vi "FW Simulator.vi"() -> ()   [LabVIEW 2015]
uses:
  Type/_RT Command.ctl
  Type/_RT Instrument State.ctl
  State.ctl
  Type/_RT Instrument 2.ctl
  Type/_RT Configuration 2.ctl
  Type/RT Loop Events.ctl
  Type/_RT Parameter.ctl
  Type/_RT Active Ch.ctl
  Type/_RT Expt.ctl
  Type/_Run Mode.ctl
  Type/_RT Mass Range.ctl
  Type/_RT Res Type.ctl
  Type/_RT Startup Options.ctl
  Type/_File Command.ctl
  Type/TCP Packet Info.ctl
  Type/_RT Data.ctl
  RT 9607/_FW_Sim Global.vi
  <vilib>/Utility/config.llb/Read Key (Boolean).vi
  Server/_Server Global.vi
  <vilib>/Utility/config.llb/NI_LVConfig.lvlib
panel:
  in  "Tab Control":enum32{"Page 1", "Page 2"}(tab)
  out "Connected":bool
  out "Command":T1
  out "# Connections":u8
  out "Messages":string="PC Communication Established"
  out "System State":T2
  in  "Stop Button":bool
  out "Remaining Scans":i32
  out "InstrState":T3
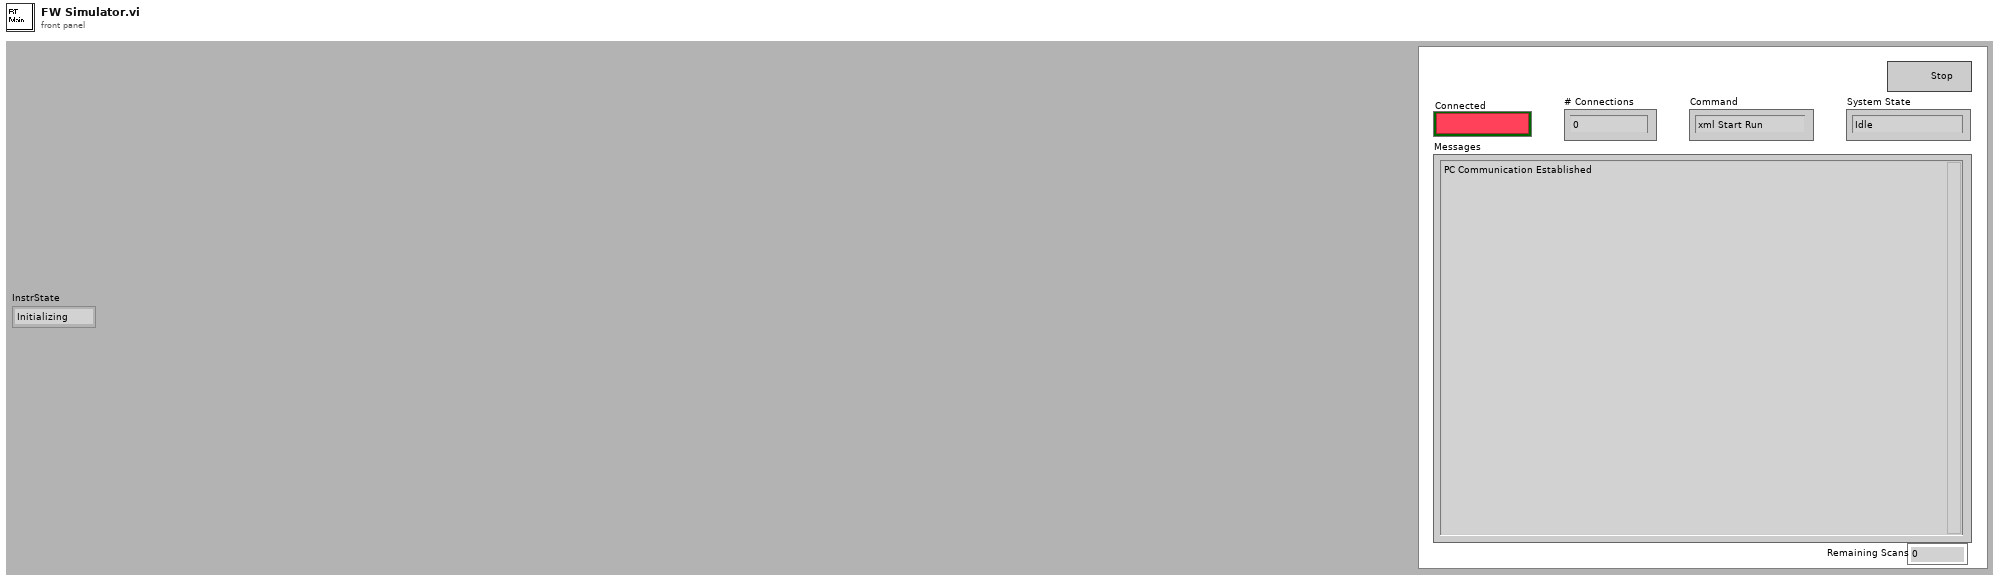
[diagram p1: front panel]
types:
  T1 = typedef "_RT Command.ctl" = enum16{"xml Start Run", "xml Start Actual Run", "xml Stop Run", "xml Runtime Update", "xml Get Status", "xml Get Table", "xml Set Table", "xml Get Configuration", "xml System Status", "xml Set LC Input Logic", "xml Get Data", "xml Get Info", "Start", "StartActualRun", "Stop", "Runtime Update", "Get Data", "Get Info", "Get Status", "Get Param", "Get Config", "Get Table", "Read ADC", "Set Oscillator", "Update Config", "Update Table", "Set All Pol", "Set Pol and DC", "Set Max Mass", "Toggle RP", "Toggle EL", "Set PIC", "Initialize Turbo", "Send Turbo Comm", "Close Turbo", "P1", "P2", "P3", "Send Serial", "Set LC Out", "Get LC In", "Read VAC", "Test Table", "Toggle Power", "Get Startup", "Set Startup", "Get ADC Table", "Set ADC Table", "Get Brief Status", "Get Detail Status", "Auxiliary Update", "Set CC Logics", "Set CC Input Logics", "Ignore Error", "invalid"}
  T2 = typedef "State.ctl" = enum16{"Idle", "Running", "Not Ready", "Fault", "Waiting"}
  T3 = typedef "_RT Instrument State.ctl" = enum16{"Initializing", "Mass Spectrometer is Off", "Starting Up", "Turning Power Off", "Going to Standby", "Roughing Pump Ready", "Turning Turbo Off", "Turbo Startup", "Turbopump Ready", "Checking Vacuum", "Going to Ready", "Ready", "Running", "Source Standby", "Lost Communication", "Shutting Down", "Fault", "24V Standby", "Go to 24V Standby", "Turbopump Ready-Waiting"}
  T4 = typedef "_RT Instrument 2.ctl" = cluster{"Table":T5[], "Instrument":string[]}
  T5 = typedef "_RT Configuration 2.ctl" = cluster{"Name":string, "Ch#":u8, "Min":dbl, "Max":dbl, "Def+":dbl, "Def-":dbl, "Offset":dbl, "Slope":dbl, "Type":u8, "Description":string, "SettleT":dbl}
  T6 = typedef "_RT Parameter.ctl" = cluster{"RunMode":i32, "Initial Ch":T7[], "Sync":u8, "Expt":T8[], "EqTime(mS)":i32}
  T7 = typedef "_RT Active Ch.ctl" = cluster{"Start":i32, "Step":i32, "ChID":i32}
  T8 = typedef "_RT Expt.ctl" = cluster{"StartT(mS)":i32, "#Cycles":i32, "Scan Type":T9, "PauseT(uS)":i32, "Polarity":u8, "DelayT(mS)":i32, "Active Ch":T7[], "Mass Range":T10[]}
  T9 = typedef "_Run Mode.ctl" = enum16{"MRM (Q1/Q2)", "Q1 Scan", "Q1 SRM", "Q2 Scan", "Q2 SRM", "Product Scan", "Precursor Scan", "Neutral Loss", "Neutral Gain"}
  T10 = typedef "_RT Mass Range.ctl" = cluster{"Steps":i32, "Dwell(uS)":i32, "Resolution Type":T11, "Ramping Ch":T7[]}
  T11 = typedef "_RT Res Type.ctl" = u16
  T12 = typedef "RT Loop Events.ctl" = enum16{"Initialize", "Wait for Connection", "Wait for Command", "Send Reply"}
  T13 = cluster{"Rt Loop Events":T12, "Connection ID":refnum<k5>, "Parameter":T6, "Message Data":string, "Data Array":i32[], "Sequence Number":i32, "Command":T1, "error":errorcluster, "Msgs":string}
  T14 = typedef "_RT Startup Options.ctl" = cluster{"Door":bool, "Curtain":bool, "Pressure":bool, "Turbo":bool, "SysPoll":bool, "GasFlag":bool}
  T15 = typedef "_File Command.ctl" = enum16{"No Command", "Open", "Open Read", "Write", "Get Spectrum", "Close"}
  T16 = enum16{"big-endian, network order", "native, host order", "little-endian"}
  T17 = typedef "TCP Packet Info.ctl" = cluster{"Packet Signature":string, "Sequence Number":i32, "Command":T1, "Data Message Size":u32, "Data Message Size":string, "Data Message":string, "Error Message Size":u32, "Error Message Size":string, "Error Message":string, "Checksum":u32, "Error Message":errorcluster, "Command ID":string}
  T18 = typedef "_RT Data.ctl" = cluster{"Info":string, "Data Array":i32[], "error out":errorcluster}
  T19 = typedef "NI_LVConfig.lvlib/Config Data RefNum.ctl" = refnum<k1>
  T20 = typedef "_XML Lens.ctl" = cluster{"Value":dbl, "ChID":u8}
  T21 = typedef "_Server Method.ctl" = cluster{"RunMode":i32, "Sync":u8, "Expt":T22[], "EqTime(mS)":i32, "TuneParam":T7[]}
  T22 = typedef "_XML Expt.ctl" = cluster{"StartT(mS)":i32, "#Cycles":i32, "PauseT(uS)":i32, "ScanType":i32, "Polarity":u8, "FixedMass":dbl, "DelayT(mS)":i32, "Active Ch":T20[], "Mass Range":T23[]}
  T23 = typedef "_Mass Range Property.ctl" = cluster{"Start":dbl, "Stop":dbl, "Step Size":dbl, "Steps":i32, "Dwell":dbl, "Parameters":T24[], "Res":T11}
  T24 = typedef "_Mass Range Parameters.ctl" = cluster{"Name":string, "Ch#":u8, "StartV":dbl, "StopV":dbl, "StepV":dbl, "Index":u8}
  T25 = enum32{"Invalid", "Standard", "Closed", "Hidden", "Minimized", "Maximized"}
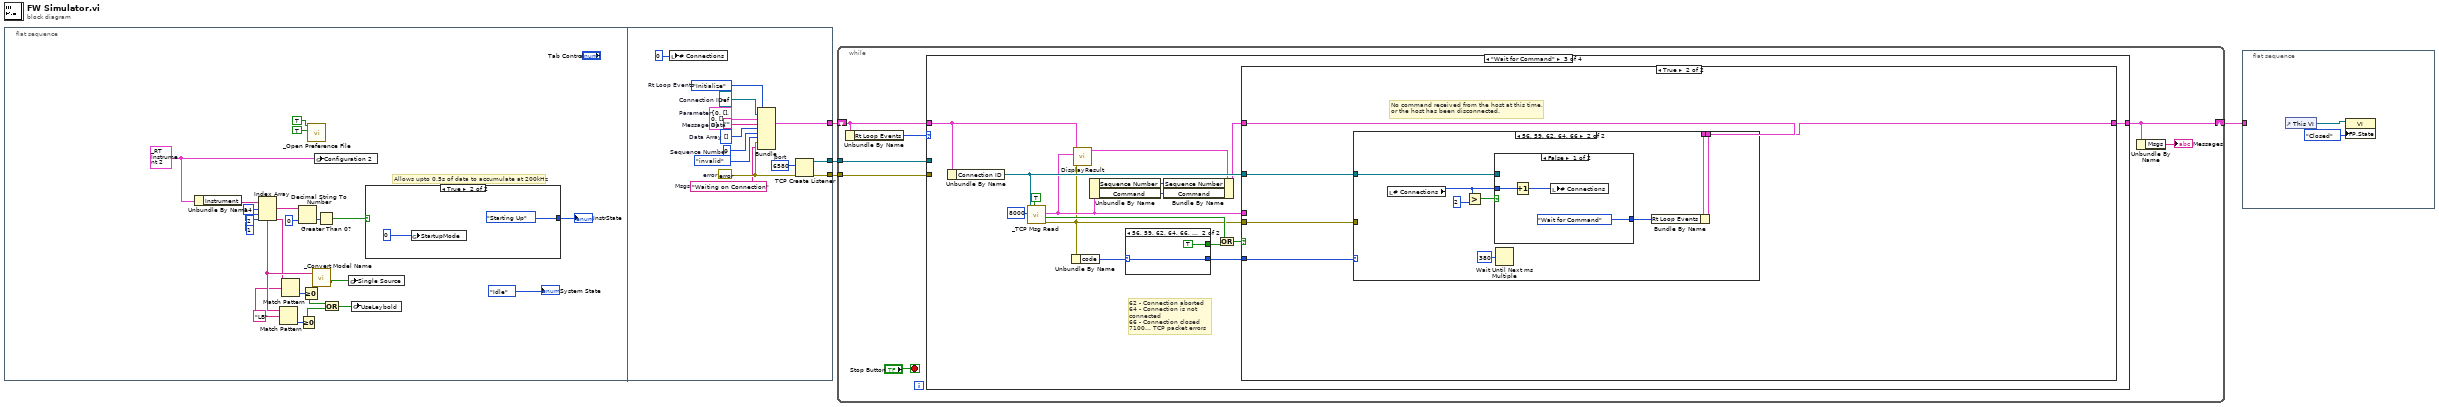
[diagram p0: block diagram]
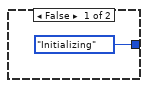
[diagram p2: hidden frame]
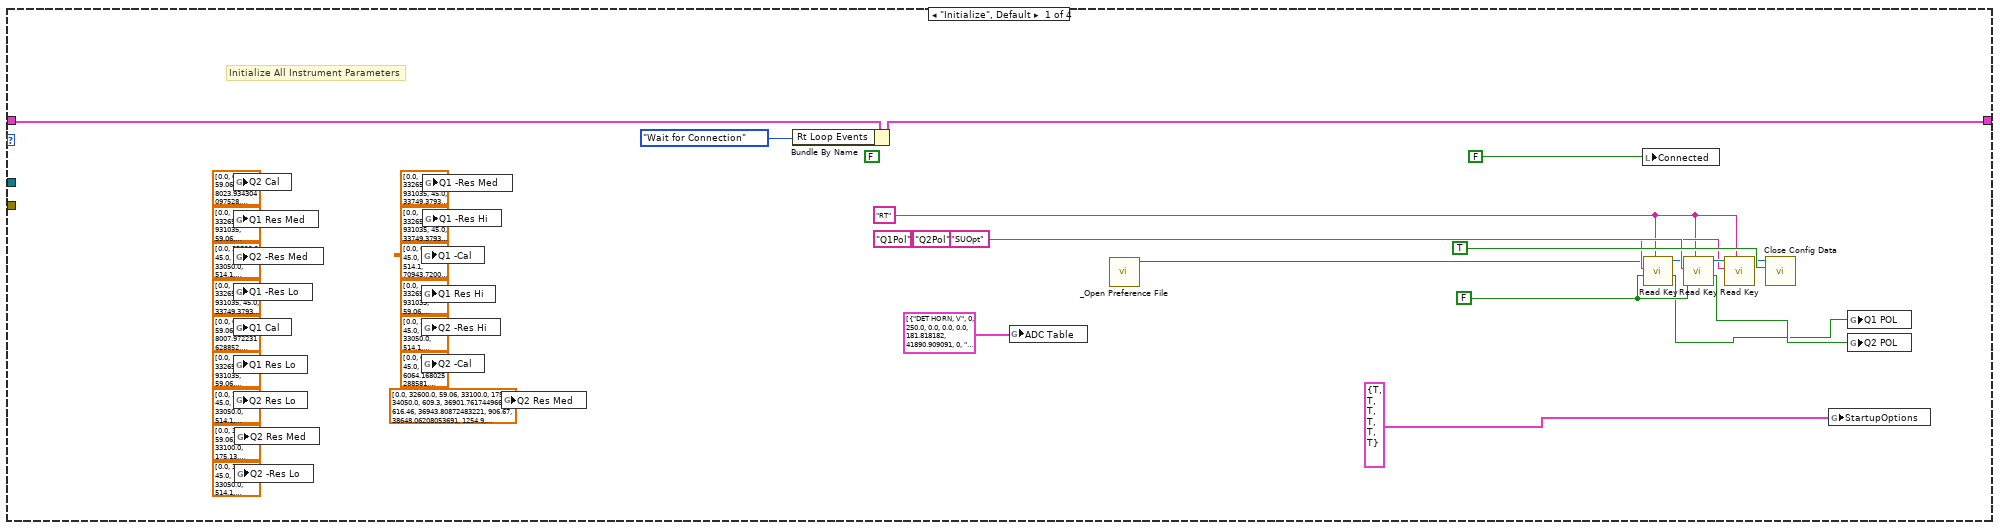
[diagram p3: hidden frame]
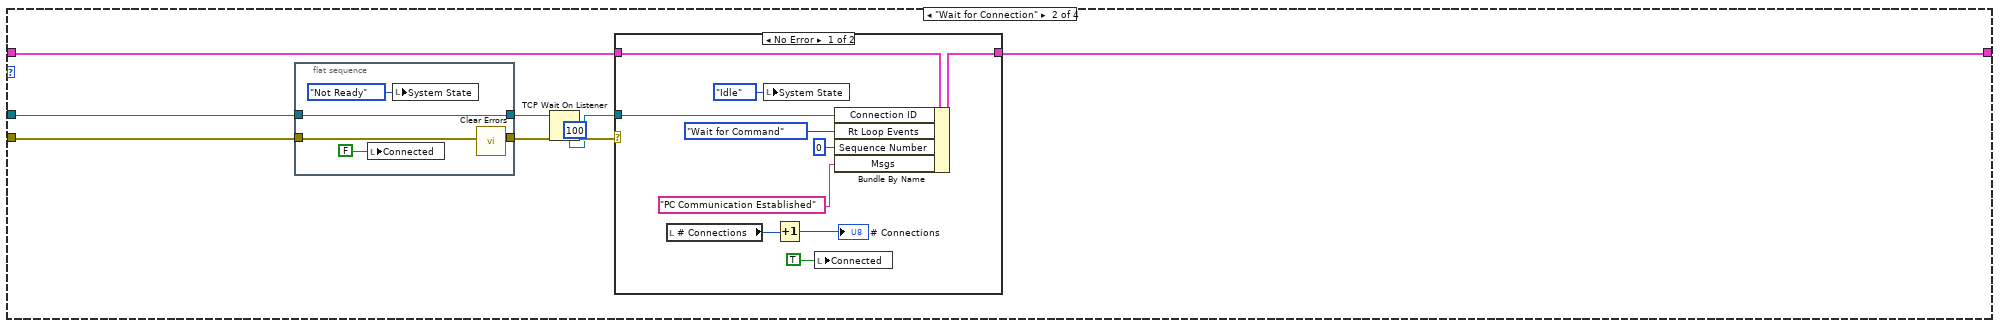
[diagram p4: hidden frame]
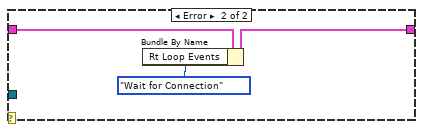
[diagram p5: hidden frame]
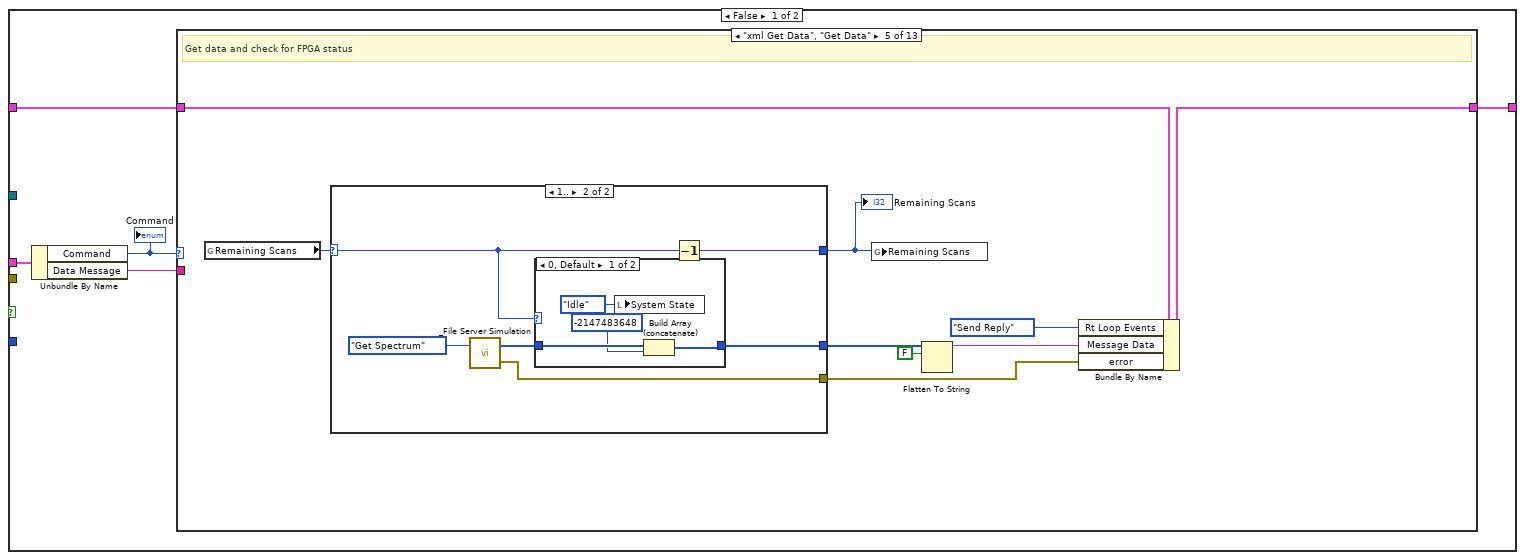
[diagram p6: hidden frame]
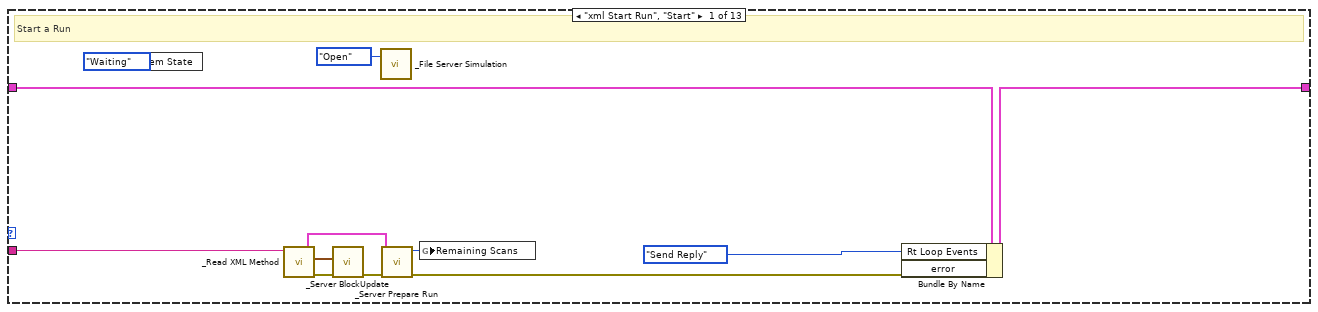
[diagram p7: hidden frame]
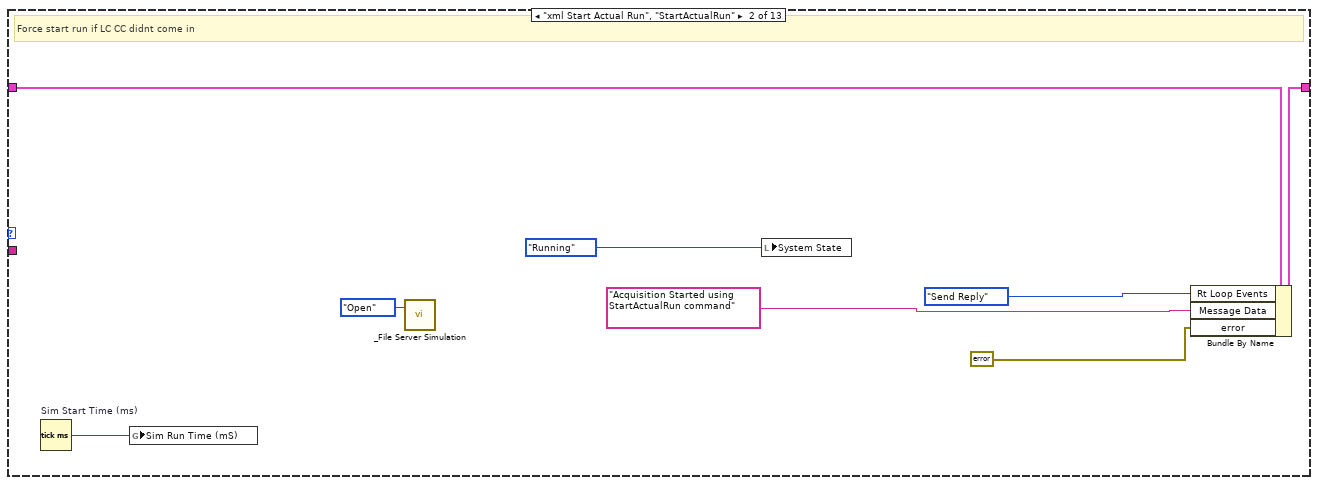
[diagram p8: hidden frame]
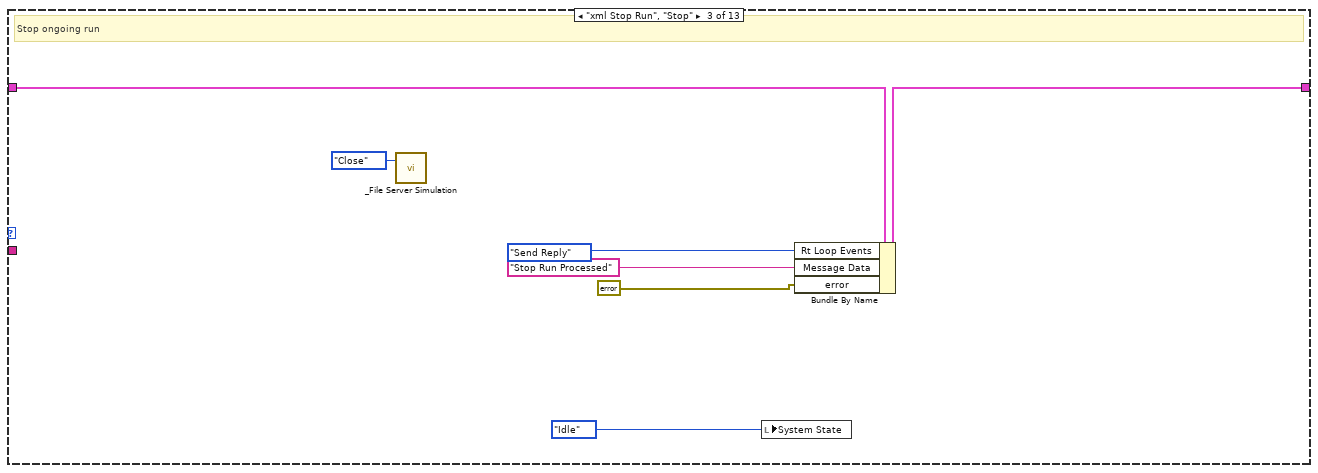
[diagram p9: hidden frame]
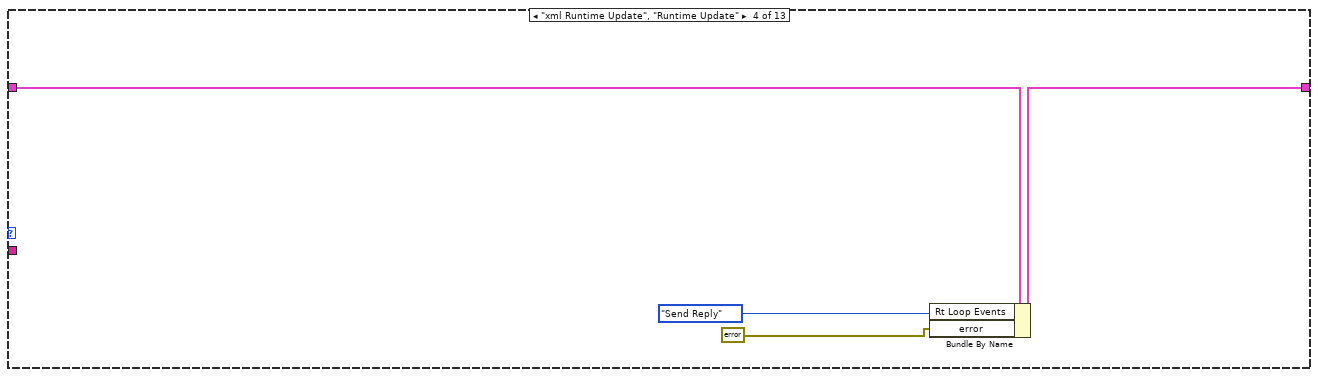
[diagram p10: hidden frame]
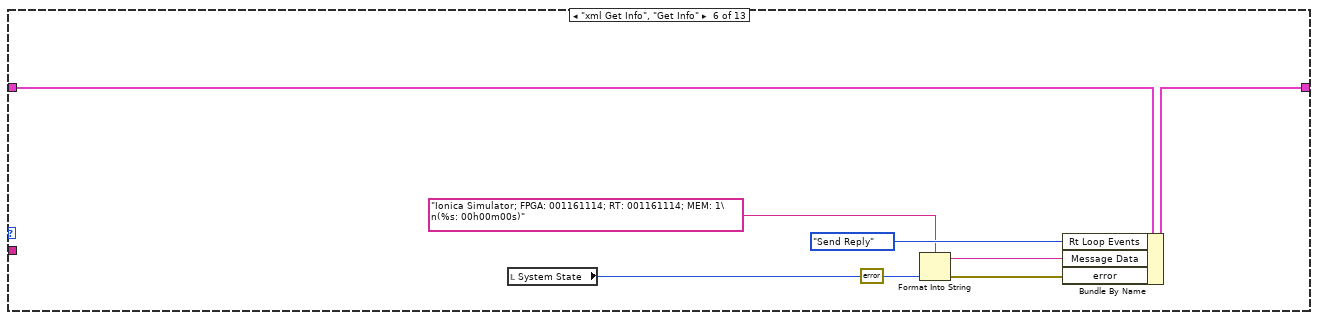
[diagram p13: hidden frame]
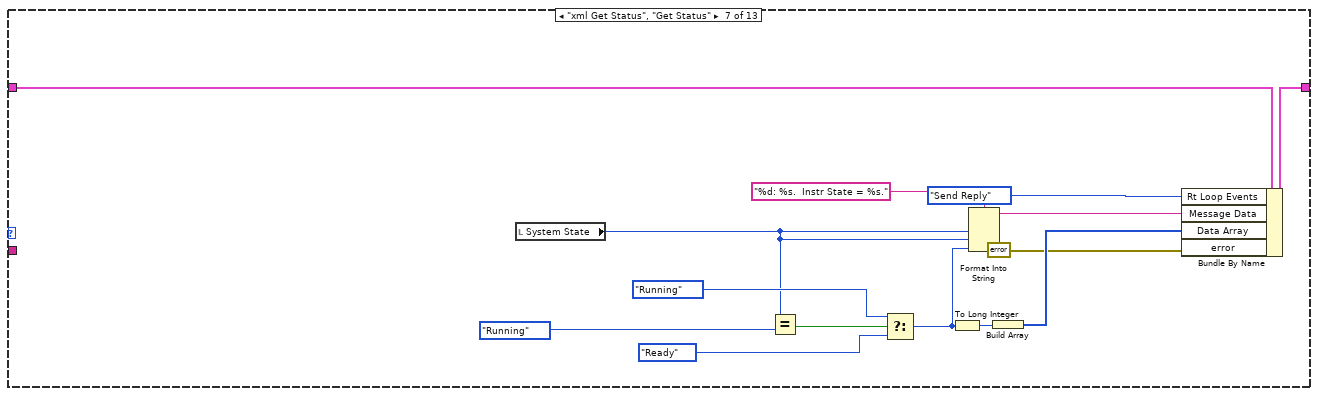
[diagram p14: hidden frame]
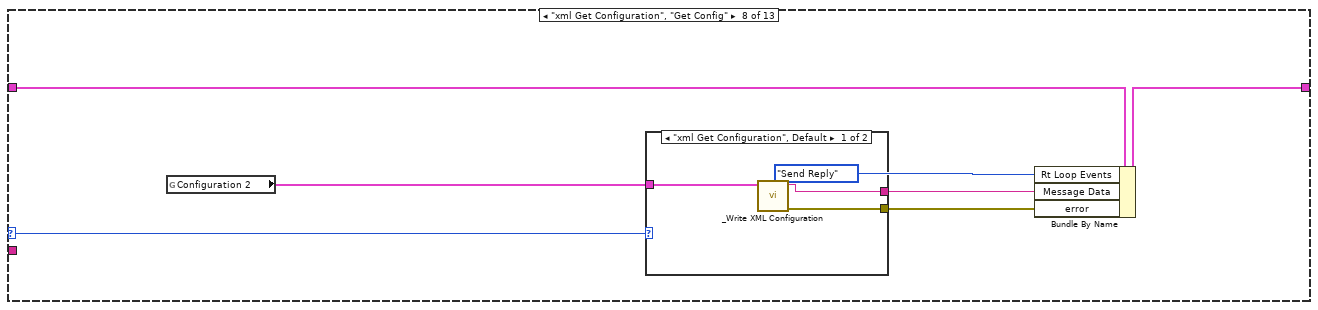
[diagram p15: hidden frame]
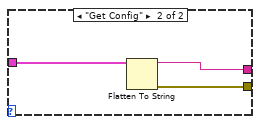
[diagram p16: hidden frame]
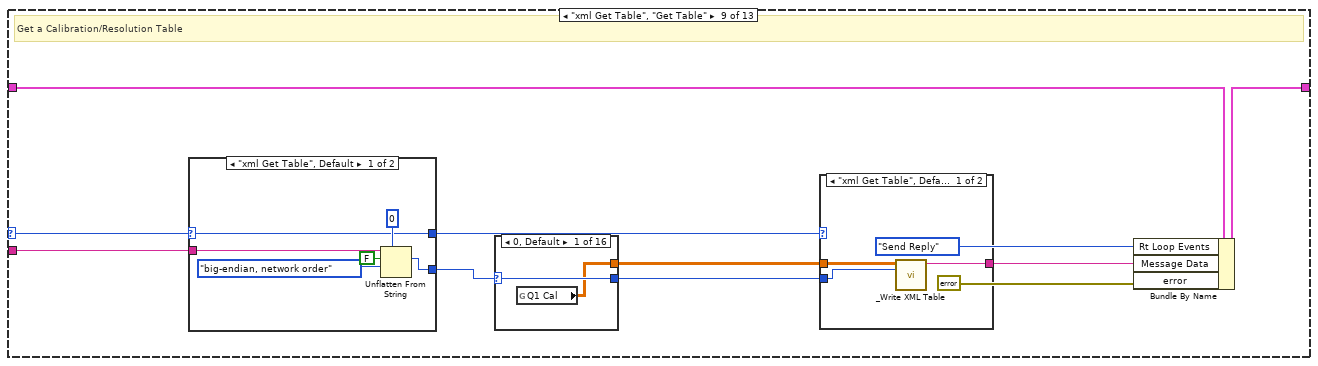
[diagram p17: hidden frame]
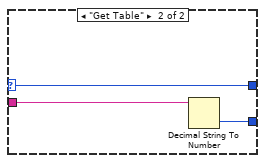
[diagram p18: hidden frame]
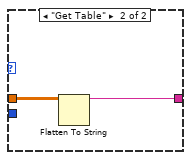
[diagram p19: hidden frame]
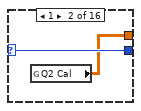
[diagram p20: hidden frame]
diagram:
  n1 = flat-sequence {
    tunnel: [w41] -> w4
    tunnel: [w37] -> w3
    tunnel: [w34] -> w2
    frame #0 {
      w5 = T4 {"Table"=[{"Name"="Q1 RF", "Ch#"=1, "Min"=0.0, "Max"=1500.0, "Def+"=0.0, "Def-"=0.0, "Offset"=0.0, "Slope"=218.45, "Type"=64, "Description"="Quadrupole 1 RF", "SettleT"=5.0}, {"Name"="Q1 DC", "Ch#"=4, "Min"=0.0, "Max"=1500.0, "Def+"=600.0, "Def-"=600.0, "Offset"=0.0, "Slope"=218.45, "Type"=64, "Description"="Quadrupole 1 DC", "SettleT"=5.0}, {"Name"="Q1 RR", "Ch#"=7, "Min"=0.0, "Max"=65535.0, "Def+"=32768.0, "Def-"=32768.0, "Offset"=32768.0, "Slope"=1.0, "Type"=64, "Description"="Quadrupole 1 PW", "SettleT"=5.0}, {"Name"="Q2 RF", "Ch#"=2, "Min"=0.0, "Max"=1500.0, "Def+"=0.0, "Def-"=0.0, "Offset"=0.0, "Slope"=218.45, "Type"=64, "Description"="Quadrupole 2 RF", "SettleT"=5.0}, {"Name"="Q2 DC", "Ch#"=5, "Min"=0.0, "Max"=1500.0, "Def+"=600.0, "Def-"=600.0, "Offset"=0.0, "Slope"=218.45, "Type"=64, "Description"="Quadrupole 2 DC", "SettleT"=5.0}, {"Name"="Q2 RR", "Ch#"=9, "Min"=0.0, "Max"=65535.0, "Def+"=32768.0, "Def-"=32768.0, "Offset"=32743.0, "Slope"=1.0, "Type"=64, "Description"="Quadrupole 2 PW", "SettleT"=5.0}, {"Name"="M1 RF", "Ch#"=3, "Min"=0.0, "Max"=500.0, "Def+"=0.0, "Def-"=0.0, "Offset"=0.0, "Slope"=14.7, "Type"=6, "Description"="Multipole 1 RF", "SettleT"=5.0}, {"Name"="EV", "Ch#"=20, "Min"=-200.0, "Max"=200.0, "Def+"=0.0, "Def-"=0.0, "Offset"=32768.0, "Slope"=-65.7, "Type"=7, "Description"="Entrance Voltage", "SettleT"=5.0}, {"Name"="ED", "Ch#"=21, "Min"=-400.0, "Max"=400.0, "Def+"=0.0, "Def-"=0.0, "Offset"=32768.0, "Slope"=-131.0, "Type"=7, "Description"="Not Used 1", "SettleT"=5.0}, {"Name"="M1", "Ch#"=19, "Min"=-400.0, "Max"=400.0, "Def+"=0.0, "Def-"=0.0, "Offset"=32775.0, "Slope"=-65.60000000000001, "Type"=7, "Description"="Multipole 1", "SettleT"=5.0}, {"Name"="L1", "Ch#"=18, "Min"=-400.0, "Max"=400.0, "Def+"=0.0, "Def-"=0.0, "Offset"=32764.0, "Slope"=-65.89999999999999, "Type"=7, "Description"="Multipole Lens 1", "SettleT"=5.0}, {"Name"="M2", "Ch#"=22, "Min"=-400.0, "Max"=400.0, "Def+"=0.0, "Def-"=0.0, "Offset"=32768.0, "Slope"=-66.0, "Type"=7, "Description"="Multipole 2", "SettleT"=5.0}, {"Name"="L2", "Ch#"=11, "Min"=-400.0, "Max"=400.0, "Def+"=0.0, "Def-"=0.0, "Offset"=32768.0, "Slope"=-65.92, "Type"=7, "Description"="Multipole Lens 2", "SettleT"=5.0}, {"Name"="PF", "Ch#"=12, "Min"=-400.0, "Max"=400.0, "Def+"=-16.0, "Def-"=16.0, "Offset"=32768.00000000001, "Slope"=-65.8, "Type"=7, "Description"="Prefilter 1", "SettleT"=5.0}, {"Name"="Q1", "Ch#"=6, "Min"=-150.0, "Max"=150.0, "Def+"=-1.0, "Def-"=1.0, "Offset"=32755.0, "Slope"=-131.3, "Type"=11, "Description"="Quadrupole 1", "SettleT"=5.0}, {"Name"="CC L1", "Ch#"=13, "Min"=-400.0, "Max"=400.0, "Def+"=0.0, "Def-"=0.0, "Offset"=32768.00000000001, "Slope"=-65.8, "Type"=7, "Description"="Collision Cell Lens 1", "SettleT"=5.0}, {"Name"="CC L2", "Ch#"=14, "Min"=-400.0, "Max"=400.0, "Def+"=-100.0, "Def-"=100.0, "Offset"=32768.00000000001, "Slope"=-65.8, "Type"=7, "Description"="Collision Cell Lens 2", "SettleT"=5.0}, {"Name"="CC", "Ch#"=23, "Min"=-400.0, "Max"=400.0, "Def+"=-50.0, "Def-"=50.0, "Offset"=32735.141073657927, "Slope"=-65.71785268414482, "Type"=7, "Description"="Collision Energy", "SettleT"=5.0}, {"Name"="CC AF", "Ch#"=10, "Min"=-400.0, "Max"=400.0, "Def+"=50.0, "Def-"=-50.0, "Offset"=32768.00000000001, "Slope"=-65.8, "Type"=7, "Description"="Axial Field", "SettleT"=5.0}, {"Name"="CC L3", "Ch#"=15, "Min"=-400.0, "Max"=400.0, "Def+"=-52.5, "Def-"=52.5, "Offset"=32735.10888610764, "Slope"=-65.7822277847309, "Type"=7, "Description"="Collision Cell Lens 3", "SettleT"=5.0}, {"Name"="CC L4", "Ch#"=16, "Min"=-400.0, "Max"=400.0, "Def+"=-72.5, "Def-"=72.5, "Offset"=32768.0, "Slope"=-65.7, "Type"=7, "Description"="Collision Cell Lens 4", "SettleT"=5.0}, {"Name"="Q2", "Ch#"=8, "Min"=-150.0, "Max"=150.0, "Def+"=-54.0, "Def-"=54.0, "Offset"=32756.0, "Slope"=-131.3, "Type"=11, "Description"="Quadrupole 2", "SettleT"=5.0}, {"Name"="ID", "Ch#"=17, "Min"=-400.0, "Max"=400.0, "Def+"=-100.0, "Def-"=100.0, "Offset"=32768.00000000001, "Slope"=-65.8, "Type"=7, "Description"="Detector Deflector", "SettleT"=5.0}, {"Name"="DISC", "Ch#"=32, "Min"=10.0, "Max"=2000.0, "Def+"=20.0, "Def-"=20.0, "Offset"=-5.0, "Slope"=1.23, "Type"=18, "Description"="Discriminator", "SettleT"=10.0}, {"Name"="DV", "Ch#"=34, "Min"=0.0, "Max"=3500.0, "Def+"=2000.0, "Def-"=2000.0, "Offset"=0.0, "Slope"=0.4104084321475626, "Type"=18, "Description"="Detector Voltage", "SettleT"=10.0}, {"Name"="DET horn", "Ch#"=200, "Min"=0.0, "Max"=5500.0, "Def+"=5500.0, "Def-"=5500.0, "Offset"=0.0, "Slope"=0.41544281263907434, "Type"=16, "Description"="Detector Horn", "SettleT"=10.0}, {"Name"="LS400A", "Ch#"=36, "Min"=0.0, "Max"=420.0, "Def+"=420.0, "Def-"=420.0, "Offset"=0.0, "Slope"=8.465116279069768, "Type"=64, "Description"="Lens Power Supply A +400", "SettleT"=5.0}, {"Name"="LS-400A", "Ch#"=37, "Min"=-420.0, "Max"=-80.0, "Def+"=-420.0, "Def-"=-420.0, "Offset"=-505.8936170212769, "Slope"=-8.553191489361703, "Type"=64, "Description"="Lens Power Supply A -400", "SettleT"=5.0}, {"Name"="LS400B", "Ch#"=38, "Min"=0.0, "Max"=420.0, "Def+"=420.0, "Def-"=420.0, "Offset"=0.0, "Slope"=8.42159383033419, "Type"=64, "Description"="Lens Power Supply B +400", "SettleT"=5.0}, {"Name"="LS-400B", "Ch#"=39, "Min"=-420.0, "Max"=-80.0, "Def+"=-420.0, "Def-"=-420.0, "Offset"=-503.5090909090908, "Slope"=-8.527272727272727, "Type"=64, "Description"="Lens Power Supply B  -400", "SettleT"=5.0}, {"Name"="QPS800", "Ch#"=40, "Min"=0.0, "Max"=600.0, "Def+"=600.0, "Def-"=600.0, "Offset"=0.0, "Slope"=4.270650263620387, "Type"=64, "Description"="Quad Power Supply +800", "SettleT"=5.0}, {"Name"="QPS-800", "Ch#"=41, "Min"=-600.0, "Max"=-140.0, "Def+"=-600.0, "Def-"=-600.0, "Offset"=-447.304347826087, "Slope"=-4.302173913043478, "Type"=64, "Description"="Quad Power Supply -800", "SettleT"=5.0}, {"Name"="DG", "Ch#"=26, "Min"=40.0, "Max"=300.0, "Def+"=80.0, "Def-"=80.0, "Offset"=0.0, "Slope"=32.765, "Type"=32, "Description"="Drying Gas", "SettleT"=1000.0}, {"Name"="NG1", "Ch#"=27, "Min"=0.0, "Max"=500.0, "Def+"=0.0, "Def-"=0.0, "Offset"=0.0, "Slope"=32.765, "Type"=32, "Description"="Nebulizer Gas 1", "SettleT"=1000.0}, {"Name"="HG1", "Ch#"=29, "Min"=0.0, "Max"=350.0, "Def+"=0.0, "Def-"=0.0, "Offset"=0.0, "Slope"=32.765, "Type"=32, "Description"="Heating Gas 1", "SettleT"=1000.0}, {"Name"="NG2", "Ch#"=28, "Min"=0.0, "Max"=500.0, "Def+"=0.0, "Def-"=0.0, "Offset"=0.0, "Slope"=32.765, "Type"=32, "Description"="Nebulizer Gas 2", "SettleT"=1000.0}, {"Name"="HG2", "Ch#"=30, "Min"=0.0, "Max"=350.0, "Def+"=0.0, "Def-"=0.0, "Offset"=0.0, "Slope"=32.765, "Type"=32, "Description"="Heating Gas 2", "SettleT"=1000.0}, {"Name"="CC P", "Ch#"=43, "Min"=0.0, "Max"=500.0, "Def+"=0.0, "Def-"=0.0, "Offset"=0.0, "Slope"=32.765, "Type"=6, "Description"="Collision Pressure", "SettleT"=3000.0}, {"Name"="SX", "Ch#"=42, "Min"=0.0, "Max"=500.0, "Def+"=0.0, "Def-"=0.0, "Offset"=0.0, "Slope"=32.765, "Type"=32, "Description"="Source Exhaust", "SettleT"=1000.0}, {"Name"="ISV2", "Ch#"=204, "Min"=-5850.0, "Max"=5850.0, "Def+"=0.0, "Def-"=0.0, "Offset"=0.0, "Slope"=0.0436, "Type"=34, "Description"="ElectroSpray V2", "SettleT"=10.0}, {"Name"="ISV1", "Ch#"=203, "Min"=-5850.0, "Max"=5850.0, "Def+"=0.0, "Def-"=0.0, "Offset"=0.0, "Slope"=0.0436, "Type"=34, "Description"="ElectroSpray V1", "SettleT"=10.0}, {"Name"="CD", "Ch#"=202, "Min"=-5.0, "Max"=5.0, "Def+"=0.0, "Def-"=0.0, "Offset"=0.0, "Slope"=51.0, "Type"=34, "Description"="Corona Discharge", "SettleT"=10.0}, {"Name"="CAP", "Ch#"=201, "Min"=-1100.0, "Max"=1100.0, "Def+"=0.0, "Def-"=0.0, "Offset"=0.0, "Slope"=0.22, "Type"=34, "Description"="Curtain Cap", "SettleT"=10.0}, {"Name"="HSID T", "Ch#"=81, "Min"=0.0, "Max"=320.0, "Def+"=320.0, "Def-"=320.0, "Offset"=0.0, "Slope"=1.0, "Type"=32, "Description"="HSID Temperature", "SettleT"=3000.0}, {"Name"="P1 T", "Ch#"=86, "Min"=0.0, "Max"=500.0, "Def+"=0.0, "Def-"=0.0, "Offset"=0.0, "Slope"=1.0, "Type"=32, "Description"="Source 1 Temp", "SettleT"=3000.0}, {"Name"="P2 T", "Ch#"=84, "Min"=0.0, "Max"=500.0, "Def+"=0.0, "Def-"=0.0, "Offset"=0.0, "Slope"=1.0, "Type"=32, "Description"="Source 2 Temp", "SettleT"=3000.0}], "Instrument"=["C:\\Users\\Public\\3Q Service\\Current\\My Configuration.c3n", "210BC608300000P", "QSight 210", "10", "20", "3000", "3000", "172.16.0.2", "F", "0", "2864776525 47914655", "2864776525 47914655", "2864776499 65665755", "0", "1", "1"]} ("Configuration 2")
      w13 = "LB" ("regular expression")
      # "Allows upto 0.5s of data to accumulate at 200kHz"
      n2 = Unbundle By Name(w5) -> ("Instrument"=w25:string[])
      n3 = Index Array(array=w25, index #1=14 ("index"), index #2=2 ("index"), index #3=1 ("index")) -> (element #1=w22:string, element #2=w17:string, element #3=w14:string)
      n4 = Match Pattern(string=w17, regular expression=w13) -> (offset past match=w18:i32)  [unwired: 4 out]
      n5 = Match Pattern(string=w14, regular expression=w13) -> (offset past match=w15:i32)  [unwired: 4 out]
      n6 = Decimal String To Number(string=w22, default (0L)=0 ("default (0 I32)")) -> (number=w21:i32)  [unwired: 2 out]
      n7 = Greater Or Equal To 0?(x=w18) -> (x >= 0?=w12:bool)
      n8 = Greater Or Equal To 0?(x=w15) -> (x >= 0?=w11:bool)
      n9 = call "_Open Preference File.vi"("Initialize"=TRUE, "Server"=TRUE) -> ()  [unwired: 1 in, 5 out]
      n10 = call "_Convert Model Name.vi"("Model"=w17) -> ("SingleSource"=w6:bool)  [unwired: 1 in, 1 out]
      n11 = global write "_FW_Sim Global.vi" "Configuration 2"(w5) -> ()
      n12 = Greater Than 0?(x=w21) -> (x > 0?=w20:bool)
      n13 = Or(x=w11, y=w12) -> (x .or. y?=w7:bool)
      n14 = global write "_FW_Sim Global.vi" "Single Source"(w6) -> ()
      n15 = global write "_FW_Sim Global.vi" "UseLeybold"(w7) -> ()
      n16 = case shown="True" w20 {
        tunnel: [_RT_Instrument_State."Initializing" ("InstrState") _RT_Instrument_State."Starting Up" ("InstrState")] -> w26
        frame False {
        }
        frame True {
          n17 = global write "_FW_Sim Global.vi" "StartupMode"(u8 0 ("StartupMode")) -> ()
        }
      }
      "InstrState" <- w26
      "System State" <- State."Idle"
    }
    frame #1 {
      w30 = "Waiting on Connection"  # Msgs
      w35 = 0  # Sequence Number
      w36 = T6 {"RunMode"=0, "Initial Ch"=[], "Sync"=0, "Expt"=[], "EqTime(mS)"=0}  # Parameter
      w38 = u16 6580  # port
      w39 = i32[] []  # Data Array
      w40 = ""  # Message Data
      w31 = errorcluster {"status"=FALSE, "code"=0, "source"=""}  # error
      w42 = refnum<k5> refnum  # Connection ID
      w43 = RT_Loop_Events."Initialize"  # Rt Loop Events
      n18 = local write "# Connections"(u8 0 ("Disconnection#")) -> ()
      n19 = Bundle("Rt Loop Events"=w43, "Connection ID"=w42, "Parameter"=w36, "Message Data"=w40, "Data Array"=w39, "Sequence Number"=w35, "Command"=_RT_Command."invalid", "error"=w31, "Msgs"=w30) -> (w41:T13)  [unwired: 1 out]
      n20 = TCP Create Listener(8:w31, 10:w38) -> (0:w34:errorcluster, 3:w37:refnum<k5>)  [unwired: 4 out]
    }
  }
  n21 = while {
    shift-right: [w46] -> w1
    shift-left: w4 -> [w49]
    tunnel: w3 -> [w48]
    tunnel: w2 -> [w47]
    stop <- "Stop Button" stop-if-true
    n22 = Unbundle By Name(w49) -> ("Rt Loop Events"=w50:T12)
    n23 = case shown="\"Wait for Command\"" w50 {
      tunnel: w49 -> [w83 w93 w115 w390]
      tunnel: [w82 w92 w126 w404] -> w46
      tunnel: w48 -> [_ w85 _ _]
      tunnel: w47 -> [_ w88 _ _]
      frame "Initialize", Default {
        (unwired) FALSE ("Connected?")
        w77 = FALSE ("Connected?")
        w74 = "RT" ("section")
        # "Initialize All Instrument Parameters"
        n24 = global write "_FW_Sim Global.vi" "Q2 Cal"(dbl[][] [[0.0, 0.0], [59.06, 8023.934304097528], [175.13, 24094.827090057508], [609.3, 84237.75059685535], [616.46, 85258.85953842459], [906.67, 125438.18017005036], [1254.9, 173704.72880677812], [1487.0, 205896.72157687077], [1500.0, 207852.79226600614]] ("Q2 Cal")) -> ()
        n25 = global write "_FW_Sim Global.vi" "Q1 Res Med"(dbl[][] [[0.0, 33265.24137931035], [59.06, 33900.54299922501], [175.13, 34950.975], [609.3, 38001.81208053691], [616.46, 38045.06040268456], [906.67, 39798.0067114094], [1254.9, 41899.39655117602], [1487.09, 43401.38461538462], [1500.0, 43600.0]] ("Q1 Res Med")) -> ()
        n26 = global write "_FW_Sim Global.vi" "Q2 -Res Med"(dbl[][] [[0.0, 32500.0], [45.0, 33050.0], [514.1, 36000.77464788732], [585.4, 36552.29226361032], [933.6, 38547.70773638968], [1223.8, 40148.896492931395], [1456.0, 41430.06819957849], [1500.0, 41672.83975467096]] ("Q2 -Res Med")) -> ()
        n27 = global write "_FW_Sim Global.vi" "Q1 -Res Lo"(dbl[][] [[0.0, 33265.24137931035], [45.0, 33749.379310344826], [514.1, 37400.0], [585.4, 37795.114503816796], [933.6, 39960.51724137931], [1223.8, 41711.724137931036], [1456.0, 43201.15291898124], [1500.0, 43600.0]] ("Q1 -Res Lo")) -> ()
        n28 = global write "_FW_Sim Global.vi" "Q1 Cal"(dbl[][] [[0.0, 0.0], [59.06, 8007.972231628852], [175.13, 24051.118700948115], [609.3, 84085.25564675158], [616.46, 85075.93195639057], [906.67, 125230.14589777726], [1254.9, 173425.601618889], [1487.09, 205562.74183429], [1500.0, 207349.59949474406]] ("Q1 Cal")) -> ()
        n29 = global write "_FW_Sim Global.vi" "Q1 Res Lo"(dbl[][] [[0.0, 33265.24137931035], [59.06, 33900.54299922501], [175.13, 34950.975], [609.3, 38001.81208053691], [616.46, 38045.06040268456], [906.67, 39798.0067114094], [1254.9, 41899.39655117602], [1487.09, 43401.38461538462], [1500.0, 43600.0]] ("Q1 Res Lo")) -> ()
        n30 = global write "_FW_Sim Global.vi" "Q2 Res Lo"(dbl[][] [[0.0, 32500.0], [45.0, 33050.0], [514.1, 36000.77464788732], [585.4, 36552.29226361032], [933.6, 38547.70773638968], [1223.8, 40148.896492931395], [1456.0, 41430.06819957849], [1500.0, 41672.83975467096]] ("Q2 Res Lo")) -> ()
        n31 = global write "_FW_Sim Global.vi" "Q2 Res Med"(dbl[][] [[0.0, 32600.0], [59.06, 33100.0], [175.13, 34050.0], [609.3, 36901.76174496644], [616.46, 36943.80872483221], [906.67, 38648.06208053691], [1254.9, 40749.39656707161], [1487.0, 42150.0], [1500.0, 42300.0]] ("Q2 Res Med")) -> ()
        n32 = global write "_FW_Sim Global.vi" "Q2 -Res Lo"(dbl[][] [[0.0, 32500.0], [45.0, 33050.0], [514.1, 36000.77464788732], [585.4, 36552.29226361032], [933.6, 38547.70773638968], [1223.8, 40148.896492931395], [1456.0, 41430.06819957849], [1500.0, 41672.83975467096]] ("Q2 -Res Lo")) -> ()
        n33 = global write "_FW_Sim Global.vi" "Q1 -Cal"(dbl[][] [[0.0, 0.0], [45.0, 6058.0], [514.1, 70943.72007379876], [585.4, 80765.52138069598], [933.6, 128993.0], [1223.8, 169105.4900068918], [1456.0, 201276.0], [1500.0, 207372.04840524014]] ("Q1 -Cal")) -> ()
        n34 = global write "_FW_Sim Global.vi" "Q1 Res Hi"(dbl[][] [[0.0, 33265.24137931035], [59.06, 33900.54299922501], [175.13, 34950.975], [609.3, 38001.81208053691], [616.46, 38045.06040268456], [906.67, 39798.0067114094], [1254.9, 41899.39655117602], [1487.09, 43401.38461538462], [1500.0, 43600.0]] ("Q1 Res Hi")) -> ()
        n35 = global write "_FW_Sim Global.vi" "Q2 -Res Hi"(dbl[][] [[0.0, 32500.0], [45.0, 33050.0], [514.1, 36000.77464788732], [585.4, 36552.29226361032], [933.6, 38547.70773638968], [1223.8, 40148.896492931395], [1456.0, 41430.06819957849], [1500.0, 41672.83975467096]] ("Q2 -Res Hi")) -> ()
        n36 = global write "_FW_Sim Global.vi" "Q2 -Cal"(dbl[][] [[0.0, 0.0], [45.0, 6064.168025288581], [514.1, 71104.0], [585.4, 80965.0], [933.6, 129151.03618609994], [1223.8, 169370.96671193905], [1456.0, 201691.0], [1500.0, 207815.38184614418]] ("Q2 -Cal")) -> ()
        n37 = global write "_FW_Sim Global.vi" "Q1 -Res Med"(dbl[][] [[0.0, 33265.24137931035], [45.0, 33749.379310344826], [514.1, 37400.0], [585.4, 37795.114503816796], [933.6, 39960.51724137931], [1223.8, 41711.724137931036], [1456.0, 43201.15291898124], [1500.0, 43600.0]] ("Q1 -Res Med")) -> ()
        n38 = global write "_FW_Sim Global.vi" "Q1 -Res Hi"(dbl[][] [[0.0, 33265.24137931035], [45.0, 33749.379310344826], [514.1, 37400.0], [585.4, 37795.114503816796], [933.6, 39960.51724137931], [1223.8, 41711.724137931036], [1456.0, 43201.15291898124], [1500.0, 43600.0]] ("Q1 -Res Hi")) -> ()
        n39 = global write "_FW_Sim Global.vi" "Q2 Res Med"(dbl[][] [[0.0, 32600.0], [59.06, 33100.0], [175.13, 34050.0], [609.3, 36901.76174496644], [616.46, 36943.80872483221], [906.67, 38648.06208053691], [1254.9, 40749.39656707161], [1487.0, 42150.0], [1500.0, 42300.0]] ("Q2 Res Med")) -> ()
        n40 = Bundle By Name(cluster=w83, "Rt Loop Events"=RT_Loop_Events."Wait for Connection") -> (w82:T13)
        n41 = global write "_FW_Sim Global.vi" "ADC Table"(T5[] [{"Name"="DET HORN, V", "Ch#"=0, "Min"=250.0, "Max"=0.0, "Def+"=0.0, "Def-"=0.0, "Offset"=181.818182, "Slope"=41890.909091, "Type"=0, "Description"="", "SettleT"=0.0}, {"Name"="DET BIAS, V", "Ch#"=0, "Min"=250.0, "Max"=0.0, "Def+"=0.0, "Def-"=0.0, "Offset"=100.0, "Slope"=40960.0, "Type"=0, "Description"="", "SettleT"=0.0}, {"Name"="Discriminator", "Ch#"=0, "Min"=5.0, "Max"=0.0, "Def+"=0.0, "Def-"=0.0, "Offset"=1.818182, "Slope"=1042.618182, "Type"=0, "Description"="", "SettleT"=0.0}, {"Name"="HED, V", "Ch#"=0, "Min"=250.0, "Max"=0.0, "Def+"=0.0, "Def-"=0.0, "Offset"=0.0, "Slope"=2015.546289, "Type"=0, "Description"="", "SettleT"=0.0}, {"Name"="DET Spare5", "Ch#"=0, "Min"=0.0, "Max"=0.0, "Def+"=0.0, "Def-"=0.0, "Offset"=0.0, "Slope"=1.0, "Type"=0, "Description"="", "SettleT"=0.0}, {"Name"="DET Spare6", "Ch#"=0, "Min"=0.0, "Max"=0.0, "Def+"=0.0, "Def-"=0.0, "Offset"=0.0, "Slope"=1.0, "Type"=0, "Description"="", "SettleT"=0.0}, {"Name"="DET Spare7", "Ch#"=0, "Min"=0.0, "Max"=0.0, "Def+"=0.0, "Def-"=0.0, "Offset"=0.0, "Slope"=1.0, "Type"=0, "Description"="", "SettleT"=0.0}, {"Name"="DET Spare8", "Ch#"=0, "Min"=0.0, "Max"=0.0, "Def+"=0.0, "Def-"=0.0, "Offset"=0.0, "Slope"=1.0, "Type"=0, "Description"="", "SettleT"=0.0}, {"Name"="Main SystemCUR (A)", "Ch#"=0, "Min"=0.0, "Max"=0.0, "Def+"=0.0, "Def-"=0.0, "Offset"=0.0, "Slope"=3.0, "Type"=0, "Description"="", "SettleT"=0.0}, {"Name"="AC Box Spare", "Ch#"=0, "Min"=0.0, "Max"=0.0, "Def+"=0.0, "Def-"=0.0, "Offset"=0.0, "Slope"=1.0, "Type"=0, "Description"="", "SettleT"=0.0}, {"Name"="+15V PS CUR (A)", "Ch#"=0, "Min"=0.0, "Max"=0.0, "Def+"=0.0, "Def-"=0.0, "Offset"=-13.5, "Slope"=5.4, "Type"=0, "Description"="", "SettleT"=0.0}, {"Name"="-15V PS CUR (A)", "Ch#"=0, "Min"=0.0, "Max"=0.0, "Def+"=0.0, "Def-"=0.0, "Offset"=-13.5, "Slope"=5.4, "Type"=0, "Description"="", "SettleT"=0.0}, {"Name"="+28V PS CUR (A)", "Ch#"=0, "Min"=0.0, "Max"=0.0, "Def+"=0.0, "Def-"=0.0, "Offset"=-25.0, "Slope"=10.0, "Type"=0, "Description"="", "SettleT"=0.0}, {"Name"="-28V PS CUR (A)", "Ch#"=0, "Min"=0.0, "Max"=0.0, "Def+"=0.0, "Def-"=0.0, "Offset"=-25.0, "Slope"=10.0, "Type"=0, "Description"="", "SettleT"=0.0}, {"Name"="+58V PS CUR (A)", "Ch#"=0, "Min"=0.0, "Max"=0.0, "Def+"=0.0, "Def-"=0.0, "Offset"=-25.0, "Slope"=10.0, "Type"=0, "Description"="", "SettleT"=0.0}, {"Name"="+24V PS CUR (A)", "Ch#"=0, "Min"=0.0, "Max"=0.0, "Def+"=0.0, "Def-"=0.0, "Offset"=-25.0, "Slope"=10.0, "Type"=0, "Description"="", "SettleT"=0.0}, {"Name"="Q1 DC POLE A, V", "Ch#"=0, "Min"=5.0, "Max"=0.0, "Def+"=0.0, "Def-"=0.0, "Offset"=0.490196, "Slope"=200.784314, "Type"=0, "Description"="", "SettleT"=0.0}, {"Name"="Q1 DC POLE B, V", "Ch#"=0, "Min"=5.0, "Max"=0.0, "Def+"=0.0, "Def-"=0.0, "Offset"=0.487805, "Slope"=199.804878, "Type"=0, "Description"="", "SettleT"=0.0}, {"Name"="Q2 DC POLE A, V", "Ch#"=0, "Min"=5.0, "Max"=0.0, "Def+"=0.0, "Def-"=0.0, "Offset"=0.492611, "Slope"=201.773399, "Type"=0, "Description"="", "SettleT"=0.0}, {"Name"="Q2 DC POLE B, V", "Ch#"=0, "Min"=5.0, "Max"=0.0, "Def+"=0.0, "Def-"=0.0, "Offset"=0.487805, "Slope"=199.804878, "Type"=0, "Description"="", "SettleT"=0.0}, {"Name"="Quad DC PS +600 V", "Ch#"=0, "Min"=10.0, "Max"=0.0, "Def+"=0.0, "Def-"=0.0, "Offset"=0.103181, "Slope"=200.749785, "Type"=0, "Description"="", "SettleT"=0.0}, {"Name"="Quad DC PS -600 V", "Ch#"=0, "Min"=10.0, "Max"=0.0, "Def+"=0.0, "Def-"=0.0, "Offset"=-1.901709, "Slope"=201.299145, "Type"=0, "Description"="", "SettleT"=0.0}, {"Name"="QDC PS +CUR (A)", "Ch#"=0, "Min"=0.0, "Max"=0.0, "Def+"=0.0, "Def-"=0.0, "Offset"=0.0, "Slope"=0.0046, "Type"=0, "Description"="", "SettleT"=0.0}, {"Name"="QDC PS -CUR (A)", "Ch#"=0, "Min"=0.0, "Max"=0.0, "Def+"=0.0, "Def-"=0.0, "Offset"=0.0, "Slope"=0.0046, "Type"=0, "Description"="", "SettleT"=0.0}, {"Name"="Q2 RF Pk-Pk, V", "Ch#"=0, "Min"=0.0, "Max"=0.0, "Def+"=0.0, "Def-"=0.0, "Offset"=0.0, "Slope"=-1208.0, "Type"=0, "Description"="", "SettleT"=0.0}, {"Name"="Q2 RF HS1 TEMP, C", "Ch#"=0, "Min"=0.0, "Max"=0.0, "Def+"=0.0, "Def-"=0.0, "Offset"=0.0, "Slope"=100.0, "Type"=0, "Description"="", "SettleT"=0.0}, {"Name"="Q2 RF HS2 TEMP, C", "Ch#"=0, "Min"=0.0, "Max"=0.0, "Def+"=0.0, "Def-"=0.0, "Offset"=0.0, "Slope"=100.0, "Type"=0, "Description"="", "SettleT"=0.0}, {"Name"="Q2 TUNING DC, V", "Ch#"=0, "Min"=0.2, "Max"=0.0, "Def+"=0.0, "Def-"=0.0, "Offset"=0.0, "Slope"=3.0, "Type"=0, "Description"="", "SettleT"=0.0}, {"Name"="Q2 RF Spare5", "Ch#"=0, "Min"=0.0, "Max"=0.0, "Def+"=0.0, "Def-"=0.0, "Offset"=0.0, "Slope"=1.0, "Type"=0, "Description"="", "SettleT"=0.0}, {"Name"="Q2 RF Spare6", "Ch#"=0, "Min"=0.0, "Max"=0.0, "Def+"=0.0, "Def-"=0.0, "Offset"=0.0, "Slope"=1.0, "Type"=0, "Description"="", "SettleT"=0.0}, {"Name"="Q2 RF Spare7", "Ch#"=0, "Min"=0.0, "Max"=0.0, "Def+"=0.0, "Def-"=0.0, "Offset"=0.0, "Slope"=1.0, "Type"=0, "Description"="", "SettleT"=0.0}, {"Name"="Q2 RF Spare8", "Ch#"=0, "Min"=0.0, "Max"=0.0, "Def+"=0.0, "Def-"=0.0, "Offset"=0.0, "Slope"=1.0, "Type"=0, "Description"="", "SettleT"=0.0}, {"Name"="CC AF +/-400, V", "Ch#"=0, "Min"=10.0, "Max"=0.0, "Def+"=0.0, "Def-"=0.0, "Offset"=0.370714, "Slope"=101.229534, "Type"=0, "Description"="", "SettleT"=0.0}, {"Name"="L2 +/-400, V", "Ch#"=0, "Min"=5.0, "Max"=0.0, "Def+"=0.0, "Def-"=0.0, "Offset"=-0.246, "Slope"=100.886703, "Type"=0, "Description"="", "SettleT"=0.0}, {"Name"="PF +/-400, V", "Ch#"=0, "Min"=10.0, "Max"=0.0, "Def+"=0.0, "Def-"=0.0, "Offset"=0.248447, "Slope"=101.763975, "Type"=0, "Description"="", "SettleT"=0.0}, {"Name"="CC L1 +/-400, V", "Ch#"=0, "Min"=10.0, "Max"=0.0, "Def+"=0.0, "Def-"=0.0, "Offset"=0.247372, "Slope"=101.323438, "Type"=0, "Description"="", "SettleT"=0.0}, {"Name"="CC L2 +/-400, V", "Ch#"=0, "Min"=10.0, "Max"=0.0, "Def+"=0.0, "Def-"=0.0, "Offset"=0.123495, "Slope"=101.167027, "Type"=0, "Description"="", "SettleT"=0.0}, {"Name"="CC L3 +/-400, V", "Ch#"=0, "Min"=10.0, "Max"=0.0, "Def+"=0.0, "Def-"=0.0, "Offset"=-0.123571, "Slope"=101.229534, "Type"=0, "Description"="", "SettleT"=0.0}, {"Name"="CC L4 +/-400, V", "Ch#"=0, "Min"=10.0, "Max"=0.0, "Def+"=0.0, "Def-"=0.0, "Offset"=0.124727, "Slope"=102.176489, "Type"=0, "Description"="", "SettleT"=0.0}, {"Name"="ID +/-400, V", "Ch#"=0, "Min"=10.0, "Max"=0.0, "Def+"=0.0, "Def-"=0.0, "Offset"=0.371402, "Slope"=101.417518, "Type"=0, "Description"="", "SettleT"=0.0}, {"Name"="L1 +/-400, V", "Ch#"=0, "Min"=5.0, "Max"=0.0, "Def+"=0.0, "Def-"=0.0, "Offset"=0.246914, "Slope"=101.135803, "Type"=0, "Description"="", "SettleT"=0.0}, {"Name"="M1 +/-400, V", "Ch#"=0, "Min"=5.0, "Max"=0.0, "Def+"=0.0, "Def-"=0.0, "Offset"=0.248, "Slope"=101.763977, "Type"=0, "Description"="", "SettleT"=0.0}, {"Name"="EV +/-400, V", "Ch#"=0, "Min"=6.0, "Max"=0.0, "Def+"=0.0, "Def-"=0.0, "Offset"=0.375235, "Slope"=102.46404, "Type"=0, "Description"="", "SettleT"=0.0}, {"Name"="Spare +/-400, V", "Ch#"=0, "Min"=5.0, "Max"=0.0, "Def+"=0.0, "Def-"=0.0, "Offset"=1.0, "Slope"=100.0, "Type"=0, "Description"="", "SettleT"=0.0}, {"Name"="M2 +/-400, V", "Ch#"=0, "Min"=5.0, "Max"=0.0, "Def+"=0.0, "Def-"=0.0, "Offset"=0.247525, "Slope"=101.386139, "Type"=0, "Description"="", "SettleT"=0.0}, {"Name"="CC +/-400, V", "Ch#"=0, "Min"=5.0, "Max"=0.0, "Def+"=0.0, "Def-"=0.0, "Offset"=-0.247831, "Slope"=101.511772, "Type"=0, "Description"="", "SettleT"=0.0}, {"Name"="Spare +/-400, V", "Ch#"=0, "Min"=0.0, "Max"=0.0, "Def+"=0.0, "Def-"=0.0, "Offset"=0.0, "Slope"=100.0, "Type"=0, "Description"="", "SettleT"=0.0}, {"Name"="Spare +/-400, V", "Ch#"=0, "Min"=0.0, "Max"=0.0, "Def+"=0.0, "Def-"=0.0, "Offset"=-1.5, "Slope"=100.0, "Type"=0, "Description"="", "SettleT"=0.0}, {"Name"="Q1 RF Pk-Pk, V", "Ch#"=0, "Min"=0.0, "Max"=0.0, "Def+"=0.0, "Def-"=0.0, "Offset"=0.0, "Slope"=-1221.0, "Type"=0, "Description"="", "SettleT"=0.0}, {"Name"="Q1 RF HS1 TEMP, C", "Ch#"=0, "Min"=0.0, "Max"=0.0, "Def+"=0.0, "Def-"=0.0, "Offset"=0.0, "Slope"=100.0, "Type"=0, "Description"="", "SettleT"=0.0}, {"Name"="Q1 RF HS2 TEMP, C", "Ch#"=0, "Min"=0.0, "Max"=0.0, "Def+"=0.0, "Def-"=0.0, "Offset"=0.0, "Slope"=100.0, "Type"=0, "Description"="", "SettleT"=0.0}, {"Name"="Q1 TUNING DC, V", "Ch#"=0, "Min"=0.2, "Max"=0.0, "Def+"=0.0, "Def-"=0.0, "Offset"=0.0, "Slope"=3.0, "Type"=0, "Description"="", "SettleT"=0.0}, {"Name"="Q1 RF Spare5", "Ch#"=0, "Min"=0.0, "Max"=0.0, "Def+"=0.0, "Def-"=0.0, "Offset"=0.0, "Slope"=1.0, "Type"=0, "Description"="", "SettleT"=0.0}, {"Name"="Q1 RF Spare6", "Ch#"=0, "Min"=0.0, "Max"=0.0, "Def+"=0.0, "Def-"=0.0, "Offset"=0.0, "Slope"=1.0, "Type"=0, "Description"="", "SettleT"=0.0}, {"Name"="Q1 RF Spare7", "Ch#"=0, "Min"=0.0, "Max"=0.0, "Def+"=0.0, "Def-"=0.0, "Offset"=0.0, "Slope"=1.0, "Type"=0, "Description"="", "SettleT"=0.0}, {"Name"="Q1 RF Spare8", "Ch#"=0, "Min"=0.0, "Max"=0.0, "Def+"=0.0, "Def-"=0.0, "Offset"=0.0, "Slope"=1.0, "Type"=0, "Description"="", "SettleT"=0.0}, {"Name"="M1 RF Pk-Pk, V", "Ch#"=0, "Min"=15.0, "Max"=0.0, "Def+"=0.0, "Def-"=0.0, "Offset"=0.0, "Slope"=-885.0, "Type"=0, "Description"="", "SettleT"=0.0}, {"Name"="M1 RF HS1 TEMP, C", "Ch#"=0, "Min"=0.0, "Max"=0.0, "Def+"=0.0, "Def-"=0.0, "Offset"=0.0, "Slope"=100.0, "Type"=0, "Description"="", "SettleT"=0.0}, {"Name"="M1 RF HS2 TEMP, C", "Ch#"=0, "Min"=0.0, "Max"=0.0, "Def+"=0.0, "Def-"=0.0, "Offset"=0.0, "Slope"=100.0, "Type"=0, "Description"="", "SettleT"=0.0}, {"Name"="M1 TUNING DC, V", "Ch#"=0, "Min"=0.2, "Max"=0.0, "Def+"=0.0, "Def-"=0.0, "Offset"=0.0, "Slope"=3.0, "Type"=0, "Description"="", "SettleT"=0.0}, {"Name"="M1 RF Spare5", "Ch#"=0, "Min"=0.0, "Max"=0.0, "Def+"=0.0, "Def-"=0.0, "Offset"=0.0, "Slope"=1.0, "Type"=0, "Description"="", "SettleT"=0.0}, {"Name"="M1 RF Spare6", "Ch#"=0, "Min"=0.0, "Max"=0.0, "Def+"=0.0, "Def-"=0.0, "Offset"=0.0, "Slope"=1.0, "Type"=0, "Description"="", "SettleT"=0.0}, {"Name"="M1 RF Spare7", "Ch#"=0, "Min"=0.0, "Max"=0.0, "Def+"=0.0, "Def-"=0.0, "Offset"=0.0, "Slope"=1.0, "Type"=0, "Description"="", "SettleT"=0.0}, {"Name"="M1 RF Spare8", "Ch#"=0, "Min"=0.0, "Max"=0.0, "Def+"=0.0, "Def-"=0.0, "Offset"=0.0, "Slope"=1.0, "Type"=0, "Description"="", "SettleT"=0.0}, {"Name"="Drying Gas Output, V", "Ch#"=0, "Min"=15.0, "Max"=0.0, "Def+"=0.0, "Def-"=0.0, "Offset"=-14.83, "Slope"=107.610001, "Type"=0, "Description"="", "SettleT"=0.0}, {"Name"="Neb Gas 1 Out, V", "Ch#"=0, "Min"=25.0, "Max"=0.0, "Def+"=0.0, "Def-"=0.0, "Offset"=-14.83, "Slope"=107.610001, "Type"=0, "Description"="", "SettleT"=0.0}, {"Name"="Neb Gas 2 Out, V", "Ch#"=0, "Min"=25.0, "Max"=0.0, "Def+"=0.0, "Def-"=0.0, "Offset"=-14.83, "Slope"=107.610001, "Type"=0, "Description"="", "SettleT"=0.0}, {"Name"="Heater Gas 1 Out, V", "Ch#"=0, "Min"=40.0, "Max"=0.0, "Def+"=0.0, "Def-"=0.0, "Offset"=-14.83, "Slope"=107.610001, "Type"=0, "Description"="", "SettleT"=0.0}, {"Name"="Heater Gas 2 Out, V", "Ch#"=0, "Min"=40.0, "Max"=0.0, "Def+"=0.0, "Def-"=0.0, "Offset"=-14.83, "Slope"=107.610001, "Type"=0, "Description"="", "SettleT"=0.0}, {"Name"="Gas box Spare6", "Ch#"=0, "Min"=0.0, "Max"=0.0, "Def+"=0.0, "Def-"=0.0, "Offset"=0.0, "Slope"=1.0, "Type"=0, "Description"="", "SettleT"=0.0}, {"Name"="SourceExhaust on/off", "Ch#"=0, "Min"=0.0, "Max"=0.0, "Def+"=0.0, "Def-"=0.0, "Offset"=0.0, "Slope"=1.0, "Type"=0, "Description"="", "SettleT"=0.0}, {"Name"="CC Gas 0-18 V, V", "Ch#"=0, "Min"=2.0, "Max"=0.0, "Def+"=0.0, "Def-"=0.0, "Offset"=0.0, "Slope"=100.0, "Type"=0, "Description"="", "SettleT"=0.0}, {"Name"="S Exhaust reading", "Ch#"=0, "Min"=0.0, "Max"=0.0, "Def+"=0.0, "Def-"=0.0, "Offset"=0.0, "Slope"=36.0, "Type"=0, "Description"="", "SettleT"=0.0}, {"Name"="Press Spare2", "Ch#"=0, "Min"=0.0, "Max"=0.0, "Def+"=0.0, "Def-"=0.0, "Offset"=0.0, "Slope"=1.0, "Type"=0, "Description"="", "SettleT"=0.0}, {"Name"="Foreline Press, torr", "Ch#"=0, "Min"=0.0, "Max"=0.0, "Def+"=0.0, "Def-"=0.0, "Offset"=1.85, "Slope"=4.5, "Type"=0, "Description"="", "SettleT"=0.0}, {"Name"="Press Spare4", "Ch#"=0, "Min"=0.0, "Max"=0.0, "Def+"=0.0, "Def-"=0.0, "Offset"=0.0, "Slope"=1.0, "Type"=0, "Description"="", "SettleT"=0.0}, {"Name"="Drying Gas Input P (V)", "Ch#"=0, "Min"=20.0, "Max"=0.0, "Def+"=0.0, "Def-"=0.0, "Offset"=-40.898998, "Slope"=29.875, "Type"=0, "Description"="", "SettleT"=0.0}, {"Name"="Press Spare6", "Ch#"=0, "Min"=0.0, "Max"=0.0, "Def+"=0.0, "Def-"=0.0, "Offset"=0.0, "Slope"=1.0, "Type"=0, "Description"="", "SettleT"=0.0}, {"Name"="Gas Manifold Input P (V)", "Ch#"=0, "Min"=20.0, "Max"=0.0, "Def+"=0.0, "Def-"=0.0, "Offset"=-40.898998, "Slope"=29.875, "Type"=0, "Description"="", "SettleT"=0.0}, {"Name"="Press Spare8", "Ch#"=0, "Min"=0.0, "Max"=0.0, "Def+"=0.0, "Def-"=0.0, "Offset"=0.0, "Slope"=1.0, "Type"=0, "Description"="", "SettleT"=0.0}, {"Name"="AC Box Spare", "Ch#"=0, "Min"=0.0, "Max"=0.0, "Def+"=0.0, "Def-"=0.0, "Offset"=0.0, "Slope"=1.0, "Type"=0, "Description"="", "SettleT"=0.0}, {"Name"="28V (+)", "Ch#"=0, "Min"=1.0, "Max"=0.0, "Def+"=0.0, "Def-"=0.0, "Offset"=0.0, "Slope"=5.8, "Type"=0, "Description"="", "SettleT"=0.0}, {"Name"="28V (-)", "Ch#"=0, "Min"=1.0, "Max"=0.0, "Def+"=0.0, "Def-"=0.0, "Offset"=0.0, "Slope"=5.8, "Type"=0, "Description"="", "SettleT"=0.0}, {"Name"="58V (+)", "Ch#"=0, "Min"=15.0, "Max"=0.0, "Def+"=0.0, "Def-"=0.0, "Offset"=0.0, "Slope"=12.0, "Type"=0, "Description"="", "SettleT"=0.0}, {"Name"="AC Box Spare", "Ch#"=0, "Min"=0.0, "Max"=0.0, "Def+"=0.0, "Def-"=0.0, "Offset"=0.0, "Slope"=1.0, "Type"=0, "Description"="", "SettleT"=0.0}, {"Name"="24V (+)", "Ch#"=0, "Min"=1.0, "Max"=0.0, "Def+"=0.0, "Def-"=0.0, "Offset"=0.0, "Slope"=5.11, "Type"=0, "Description"="", "SettleT"=0.0}, {"Name"="15V (+)", "Ch#"=0, "Min"=1.0, "Max"=0.0, "Def+"=0.0, "Def-"=0.0, "Offset"=0.0, "Slope"=3.18, "Type"=0, "Description"="", "SettleT"=0.0}, {"Name"="15V (-)", "Ch#"=0, "Min"=1.0, "Max"=0.0, "Def+"=0.0, "Def-"=0.0, "Offset"=0.0, "Slope"=3.18, "Type"=0, "Description"="", "SettleT"=0.0}, {"Name"="LN2 PS Pos (V)", "Ch#"=0, "Min"=20.0, "Max"=0.0, "Def+"=0.0, "Def-"=0.0, "Offset"=1.111111, "Slope"=100.278719, "Type"=0, "Description"="", "SettleT"=0.0}, {"Name"="LN2 PS Neg (V)", "Ch#"=0, "Min"=20.0, "Max"=0.0, "Def+"=0.0, "Def-"=0.0, "Offset"=-2.047619, "Slope"=100.524542, "Type"=0, "Description"="", "SettleT"=0.0}, {"Name"="LN2 PS +CUR (A)", "Ch#"=0, "Min"=0.0, "Max"=0.0, "Def+"=0.0, "Def-"=0.0, "Offset"=0.0, "Slope"=0.0046, "Type"=0, "Description"="", "SettleT"=0.0}, {"Name"="LN2 PS -CUR (A)", "Ch#"=0, "Min"=0.0, "Max"=0.0, "Def+"=0.0, "Def-"=0.0, "Offset"=0.0, "Slope"=0.0046, "Type"=0, "Description"="", "SettleT"=0.0}, {"Name"="Lens Board 2 +5V", "Ch#"=0, "Min"=0.2, "Max"=0.0, "Def+"=0.0, "Def-"=0.0, "Offset"=0.0, "Slope"=1.0, "Type"=0, "Description"="", "SettleT"=0.0}, {"Name"="Lens Board 2 -5V", "Ch#"=0, "Min"=0.2, "Max"=0.0, "Def+"=0.0, "Def-"=0.0, "Offset"=0.0, "Slope"=1.0, "Type"=0, "Description"="", "SettleT"=0.0}, {"Name"="LN2 HVPS Reference", "Ch#"=0, "Min"=0.2, "Max"=0.0, "Def+"=0.0, "Def-"=0.0, "Offset"=0.0, "Slope"=1.0, "Type"=0, "Description"="", "SettleT"=0.0}, {"Name"="L1-ADC12-8", "Ch#"=0, "Min"=0.0, "Max"=0.0, "Def+"=0.0, "Def-"=0.0, "Offset"=0.0, "Slope"=1.0, "Type"=0, "Description"="", "SettleT"=0.0}, {"Name"="LN1 PS Pos (V)", "Ch#"=0, "Min"=20.0, "Max"=0.0, "Def+"=0.0, "Def-"=0.0, "Offset"=0.339409, "Slope"=100.404777, "Type"=0, "Description"="", "SettleT"=0.0}, {"Name"="LN1 PS Neg (V)", "Ch#"=0, "Min"=20.0, "Max"=0.0, "Def+"=0.0, "Def-"=0.0, "Offset"=-1.863104, "Slope"=100.450952, "Type"=0, "Description"="", "SettleT"=0.0}, {"Name"="LN1 PS +CUR (A)", "Ch#"=0, "Min"=0.0, "Max"=0.0, "Def+"=0.0, "Def-"=0.0, "Offset"=0.0, "Slope"=0.01765, "Type"=0, "Description"="", "SettleT"=0.0}, {"Name"="LN1 PS -CUR (A)", "Ch#"=0, "Min"=0.0, "Max"=0.0, "Def+"=0.0, "Def-"=0.0, "Offset"=0.0, "Slope"=0.01765, "Type"=0, "Description"="", "SettleT"=0.0}, {"Name"="Lens Board 1 +5V", "Ch#"=0, "Min"=0.2, "Max"=0.0, "Def+"=0.0, "Def-"=0.0, "Offset"=0.0, "Slope"=1.0, "Type"=0, "Description"="", "SettleT"=0.0}, {"Name"="Lens Board 1 -5V", "Ch#"=0, "Min"=0.2, "Max"=0.0, "Def+"=0.0, "Def-"=0.0, "Offset"=0.0, "Slope"=1.0, "Type"=0, "Description"="", "SettleT"=0.0}, {"Name"="LN1 HVPS Reference", "Ch#"=0, "Min"=0.2, "Max"=0.0, "Def+"=0.0, "Def-"=0.0, "Offset"=0.0, "Slope"=1.0, "Type"=0, "Description"="", "SettleT"=0.0}, {"Name"="L3-ADC13-8", "Ch#"=0, "Min"=0.0, "Max"=0.0, "Def+"=0.0, "Def-"=0.0, "Offset"=0.0, "Slope"=1.0, "Type"=0, "Description"="", "SettleT"=0.0}, {"Name"="CAP Voltage", "Ch#"=0, "Min"=150.0, "Max"=0.0, "Def+"=0.0, "Def-"=0.0, "Offset"=0.0, "Slope"=13.9, "Type"=0, "Description"="", "SettleT"=0.0}, {"Name"="HSID T", "Ch#"=0, "Min"=30.0, "Max"=0.0, "Def+"=0.0, "Def-"=0.0, "Offset"=0.0, "Slope"=1.0, "Type"=0, "Description"="", "SettleT"=0.0}, {"Name"="CD Corona", "Ch#"=0, "Min"=0.4, "Max"=0.0, "Def+"=0.0, "Def-"=0.0, "Offset"=0.0, "Slope"=0.025, "Type"=0, "Description"="", "SettleT"=0.0}, {"Name"="ISV1 Voltage", "Ch#"=0, "Min"=350.0, "Max"=0.0, "Def+"=0.0, "Def-"=0.0, "Offset"=0.0, "Slope"=24.0, "Type"=0, "Description"="", "SettleT"=0.0}, {"Name"="Probe2 Temp", "Ch#"=0, "Min"=40.0, "Max"=0.0, "Def+"=0.0, "Def-"=0.0, "Offset"=0.0, "Slope"=1.0, "Type"=0, "Description"="", "SettleT"=0.0}, {"Name"="ISV2 Voltage", "Ch#"=0, "Min"=350.0, "Max"=0.0, "Def+"=0.0, "Def-"=0.0, "Offset"=0.0, "Slope"=24.0, "Type"=0, "Description"="", "SettleT"=0.0}, {"Name"="Probe1 Temp", "Ch#"=0, "Min"=40.0, "Max"=0.0, "Def+"=0.0, "Def-"=0.0, "Offset"=0.0, "Slope"=1.0, "Type"=0, "Description"="", "SettleT"=0.0}, {"Name"="PIC 87", "Ch#"=0, "Min"=0.0, "Max"=0.0, "Def+"=0.0, "Def-"=0.0, "Offset"=0.0, "Slope"=1.0, "Type"=0, "Description"="", "SettleT"=0.0}, {"Name"="PIC 88", "Ch#"=0, "Min"=0.0, "Max"=0.0, "Def+"=0.0, "Def-"=0.0, "Offset"=0.0, "Slope"=1.0, "Type"=0, "Description"="", "SettleT"=0.0}, {"Name"="PROBE 1 ID", "Ch#"=0, "Min"=0.0, "Max"=0.0, "Def+"=0.0, "Def-"=0.0, "Offset"=0.0, "Slope"=1.0, "Type"=0, "Description"="", "SettleT"=0.0}, {"Name"="PROBE 2 ID", "Ch#"=0, "Min"=0.0, "Max"=0.0, "Def+"=0.0, "Def-"=0.0, "Offset"=0.0, "Slope"=1.0, "Type"=0, "Description"="", "SettleT"=0.0}, {"Name"="PIC Spare", "Ch#"=0, "Min"=0.0, "Max"=0.0, "Def+"=0.0, "Def-"=0.0, "Offset"=0.0, "Slope"=1.0, "Type"=0, "Description"="", "SettleT"=0.0}, {"Name"="PIC Spare", "Ch#"=0, "Min"=0.0, "Max"=0.0, "Def+"=0.0, "Def-"=0.0, "Offset"=0.0, "Slope"=1.0, "Type"=0, "Description"="", "SettleT"=0.0}, {"Name"="PIC Spare", "Ch#"=0, "Min"=0.0, "Max"=0.0, "Def+"=0.0, "Def-"=0.0, "Offset"=0.0, "Slope"=1.0, "Type"=0, "Description"="", "SettleT"=0.0}, {"Name"="PIC Spare", "Ch#"=0, "Min"=0.0, "Max"=0.0, "Def+"=0.0, "Def-"=0.0, "Offset"=0.0, "Slope"=1.0, "Type"=0, "Description"="", "SettleT"=0.0}, {"Name"="VAC Gauge", "Ch#"=0, "Min"=0.0, "Max"=0.0, "Def+"=0.0, "Def-"=0.0, "Offset"=0.0, "Slope"=1.0, "Type"=0, "Description"="", "SettleT"=0.0}, {"Name"="Door Interlock", "Ch#"=0, "Min"=0.0, "Max"=0.0, "Def+"=0.0, "Def-"=0.0, "Offset"=0.0, "Slope"=1.0, "Type"=0, "Description"="", "SettleT"=0.0}, {"Name"="Vacuum Ready", "Ch#"=0, "Min"=0.0, "Max"=0.0, "Def+"=0.0, "Def-"=0.0, "Offset"=0.0, "Slope"=1.0, "Type"=0, "Description"="", "SettleT"=0.0}, {"Name"="LC1 Out1 Hold", "Ch#"=0, "Min"=0.0, "Max"=0.0, "Def+"=0.0, "Def-"=0.0, "Offset"=0.0, "Slope"=1.0, "Type"=0, "Description"="", "SettleT"=0.0}, {"Name"="LC1 Out2 Stop", "Ch#"=0, "Min"=0.0, "Max"=0.0, "Def+"=0.0, "Def-"=0.0, "Offset"=0.0, "Slope"=1.0, "Type"=0, "Description"="", "SettleT"=0.0}, {"Name"="LC2 Out1 Hold", "Ch#"=0, "Min"=0.0, "Max"=0.0, "Def+"=0.0, "Def-"=0.0, "Offset"=0.0, "Slope"=1.0, "Type"=0, "Description"="", "SettleT"=0.0}, {"Name"="LC2 Out2 Stop", "Ch#"=0, "Min"=0.0, "Max"=0.0, "Def+"=0.0, "Def-"=0.0, "Offset"=0.0, "Slope"=1.0, "Type"=0, "Description"="", "SettleT"=0.0}, {"Name"="LC1 In", "Ch#"=0, "Min"=0.0, "Max"=0.0, "Def+"=0.0, "Def-"=0.0, "Offset"=0.0, "Slope"=1.0, "Type"=0, "Description"="", "SettleT"=0.0}, {"Name"="LC2 In", "Ch#"=0, "Min"=0.0, "Max"=0.0, "Def+"=0.0, "Def-"=0.0, "Offset"=0.0, "Slope"=1.0, "Type"=0, "Description"="", "SettleT"=0.0}] ("ADC Table")) -> ()
        n42 = call "_Open Preference File.vi"() -> ("refnum"=w69:T19)  [unwired: 3 in, 4 out]
        n43 = local write "Connected"(FALSE ("Connected?")) -> ()
        n44 = call-poly <vilib>:"Read Key.vi"("section"=w74, "default value"=w77, "key"="Q1Pol", "refnum"=w69) -> ("value"=w70:bool, "refnum out"=w78:T19)  [unwired: 1 in, 5 out]
        n45 = call-poly <vilib>:"Read Key.vi"("section"=w74, "default value"=w77, "key"="Q2Pol", "refnum"=w78) -> ("value"=w71:bool, "refnum out"=w76:T19)  [unwired: 1 in, 5 out]
        n46 = call-poly <vilib>:"Read Key.vi"("section"=w74, "key"="SUOpt", "refnum"=w76) -> ("refnum out"=w73:T19)  [unwired: 2 in, 6 out]
        n47 = call <vilib>:"Close Config Data.vi"("write file if changed (T)"=TRUE ("write configuration file? (T)"), "refnum"=w73) -> ()  [unwired: 1 in, 9 out]
        n48 = global write "_FW_Sim Global.vi" "StartupOptions"(T14 {"Door"=TRUE, "Curtain"=TRUE, "Pressure"=TRUE, "Turbo"=TRUE, "SysPoll"=TRUE, "GasFlag"=TRUE} ("StartupOptions")) -> ()
        n49 = global write "_FW_Sim Global.vi" "Q1 POL"(w70) -> ()
        n50 = global write "_FW_Sim Global.vi" "Q2 POL"(w71) -> ()
      }
      frame "Wait for Connection" {
        n51 = flat-sequence {
          tunnel: w88 -> [w98]
          tunnel: [w97] -> w87
          tunnel: [w96] -> w86
          tunnel: w85 -> [w96]
          frame #0 {
            n52 = local write "Connected"(FALSE ("Connected?")) -> ()
            n53 = local write "System State"(State."Not Ready" ("System State")) -> ()
            n54 = call <vilib>:"Clear Errors.vi"("error in (no error)"=w98) -> ("error out"=w97:errorcluster)  [unwired: 5 in, 1 out]
          }
        }
        n55 = TCP Wait On Listener(8:w87, 9:100 ("timeout ms (wait forever: -1)"), 11:w86) -> (0:w91:errorcluster, 4:w90:refnum<k5>)  [unwired: 4 out]
        n56 = case shown="No Error" w91 {
          tunnel: w93 -> [w108 w111]
          tunnel: w90 -> [w106 _]
          tunnel: [w107 w109] -> w92
          frame No Error {
            n57 = local read "# Connections"() -> (w100:u8)
            n58 = local write "System State"(State."Idle" ("System State")) -> ()
            n59 = Increment(x=w100) -> (x+1=→"# Connections":u8)
            n60 = local write "Connected"(TRUE ("Connected?")) -> ()
            n61 = Bundle By Name(cluster=w108, "Connection ID"=w106, "Rt Loop Events"=RT_Loop_Events."Wait for Command", "Sequence Number"=0, "Msgs"="PC Communication Established" ("Event")) -> (w107:T13)
          }
          frame Error {
            n62 = Bundle By Name(cluster=w111, "Rt Loop Events"=RT_Loop_Events."Wait for Connection") -> (w109:T13)
          }
        }
      }
      frame "Wait for Command" {
        # "62 - Connection aborted\n64 - Connection is not connected\n66 - Connection closed\n7100... TCP packet errors"
        n63 = Unbundle By Name(w115) -> ("Connection ID"=w123:refnum<k5>)
        n64 = call "_TCP Msg Read.vi"("RT"=TRUE, "timeout ms (10000)"=8000 ("millisecond multiple"), "connection ID"=w123) -> ("error out"=w112:errorcluster, "Read Timeout"=w120:bool, "Packet Info"=w116:T17)  [unwired: 1 in, 5 out]
        n65 = Unbundle By Name(w112) -> ("code"=w127:i32)
        n66 = call "DisplayResult.vi"("error in (no error)"=w112, "Packet Info"=w116, "Cluster"=w115) -> ("Cluster out"=w114:T13)  [unwired: 7 in, 1 out]
        n67 = Unbundle By Name(w116) -> ("Sequence Number"=w118:i32, "Command"=w117:T1)
        n68 = case shown="56, 59, 62, 64, 66, 7100.., Default" w127 {
          selector: w127 -> [w381 w382]
          tunnel: [_ TRUE ("abort (F)")] -> w122
          tunnel: [w381 w382] -> w113
          frame 0 {
          }
          frame 56, 59, 62, 64, 66, 7100.., Default {
          }
        }
        n69 = Bundle By Name(cluster=w114, "Sequence Number"=w118, "Command"=w117) -> (w119:T13)
        n70 = Or(x=w120, y=w122) -> (x .or. y?=w124:bool)
        n71 = case shown="True" w124 {
          tunnel: w119 -> [w132 w361]
          tunnel: [w131 w360] -> w126
          tunnel: w116 -> [w130 _]
          tunnel: w123 -> [_ w359]
          tunnel: w113 -> [_ w358]
          tunnel: w112 -> [_ w357]
          frame False {
            n72 = Unbundle By Name(w130) -> ("Command"=w129:T1, "Data Message"=w128:string)
            "Command" <- w129
            n73 = case shown="\"xml Get Data\", \"Get Data\"" w129 {
              selector: w129 -> [_ _ _ _ _ _ _ w207 w223 _ _ _ w352]
              tunnel: w128 -> [w134 _ _ _ _ _ _ _ w226 w282 _ _ _]
              tunnel: w132 -> [w143 w151 w159 w162 w172 w191 w205 w212 w229 w286 w341 w345 w354]
              tunnel: [w142 w150 w158 w161 w171 w190 w204 w211 w228 w284 w340 w344 w353] -> w131
              frame "xml Start Run", "Start" {
                # "Start a Run"
                n74 = local write "System State"(State."Waiting" ("System State")) -> ()
                n75 = call "_Read XML Method.vi"("XML String"=w134) -> ("error out"=w138:errorcluster, "Lens"=w137:T20[], "Server Method"=w135:T21)  [unwired: 1 in, 3 out]
                n76 = call "_Server BlockUpdate.vi"("error in"=w138, "Lens"=w137) -> ("error out"=w136:errorcluster)  [unwired: 2 in, 3 out]
                n77 = call "_File Server Simulation.vi"("FileCommand"=_File_Command."Open") -> ()  [unwired: 1 in, 2 out]
                n78 = call "_Server Prepare Run.vi"("error in (no error)"=w136, "Server Method"=w135) -> ("error out"=w133:errorcluster, "Scans"=w139:i32)  [unwired: 1 in, 7 out]
                n79 = global write "_Server Global.vi" "Remaining Scans"(w139) -> ()
                n80 = Bundle By Name(cluster=w143, "Rt Loop Events"=RT_Loop_Events."Send Reply", "error"=w133) -> (w142:T13)
              }
              frame "xml Start Actual Run", "StartActualRun" {
                # "Force start run if LC CC didnt come in"
                n81 = Tick Count (ms) "Sim Start Time (ms)"() -> (millisecond timer value=w145:u32)
                n82 = global write "_Server Global.vi" "Sim Run Time (mS)"(w145) -> ()
                n83 = call "_File Server Simulation.vi"("FileCommand"=_File_Command."Open") -> ()  [unwired: 1 in, 2 out]
                n84 = local write "System State"(State."Running" ("System State")) -> ()
                n85 = Bundle By Name(cluster=w151, "Rt Loop Events"=RT_Loop_Events."Send Reply", "Message Data"="Acquisition Started using StartActualRun command" ("source"), "error"=errorcluster {"status"=FALSE, "code"=0, "source"=""}) -> (w150:T13)
              }
              frame "xml Stop Run", "Stop" {
                # "Stop ongoing run"
                n86 = call "_File Server Simulation.vi"("FileCommand"=_File_Command."Close") -> ()  [unwired: 1 in, 2 out]
                n87 = local write "System State"(State."Idle" ("System State")) -> ()
                n88 = Bundle By Name(cluster=w159, "Rt Loop Events"=RT_Loop_Events."Send Reply", "Message Data"="Stop Run Processed" ("string"), "error"=errorcluster {"status"=FALSE, "code"=0, "source"=""}) -> (w158:T13)
              }
              frame "xml Runtime Update", "Runtime Update" {
                n89 = Bundle By Name(cluster=w162, "Rt Loop Events"=RT_Loop_Events."Send Reply", "error"=errorcluster {"status"=FALSE, "code"=0, "source"=""}) -> (w161:T13)
              }
              frame "xml Get Data", "Get Data" {
                # "Get data and check for FPGA status"
                n90 = global read "_Server Global.vi" "Remaining Scans"() -> (w166:i32)
                n91 = case shown="1.." w166 {
                  selector: w166 -> [w173 w176]
                  tunnel: [_ w179] -> w167
                  tunnel: [w173 w178] -> w164
                  tunnel: [_ w174] -> w165
                  frame Default {
                  }
                  frame 1.. {
                    n92 = call "_File Server Simulation.vi"("FileCommand"=_File_Command."Get Spectrum") -> ("ErrorOut"=w179:errorcluster, "DataArray"=w175:i32[])  [unwired: 1 in]
                    n93 = case shown="0, Default" w176 {
                      tunnel: w175 -> [w183 w184]
                      tunnel: [w181 w184] -> w174
                      frame 0, Default {
                        n94 = local write "System State"(State."Idle" ("System State")) -> ()
                        n95 = Build Array (concatenate)(w183, -2147483648) -> (w181:i32[])
                      }
                      frame 2.. {
                      }
                    }
                    n96 = Decrement(x=w176) -> (x-1=w178:i32)
                  }
                }
                "Remaining Scans" <- w164
                n97 = global write "_Server Global.vi" "Remaining Scans"(w164) -> ()
                n98 = Flatten To String(anything=w165, prepend array or string size? (T)=FALSE) -> (data string=w168:string)  [unwired: 2 in, 2 out]
                n99 = Bundle By Name(cluster=w172, "Rt Loop Events"=RT_Loop_Events."Send Reply", "Message Data"=w168, "error"=w167) -> (w171:T13)
              }
              frame "xml Get Info", "Get Info" {
                n100 = local read "System State"() -> (w186:T2)
                n101 = Format Into String(format string="Ionica Simulator; FPGA: 001161114; RT: 001161114; MEM: 1\n(%s: 00h00m00s)", w186) -> (resulting string=w187:string)  [unwired: 2 in, 1 out]
                n102 = Bundle By Name(cluster=w191, "Rt Loop Events"=RT_Loop_Events."Send Reply", "Message Data"=w187, "error"=errorcluster {"status"=FALSE, "code"=0, "source"=""}) -> (w190:T13)
              }
              frame "xml Get Status", "Get Status" {
                n103 = local read "System State"() -> (w193:T2)
                n104 = Equal?(x=w193, y=State."Running" ("System State")) -> (x = y?=w197:bool)
                n105 = Select(t=_RT_Instrument_State."Running" ("InstrState"), s=w197, f=_RT_Instrument_State."Ready" ("InstrState")) -> (s? t:f=w194:T3)
                n106 = To Long Integer(number=w194) -> (32bit integer=w202:i32)
                n107 = Format Into String(format string="%d: %s.  Instr State = %s.", w193, w193, w194) -> (resulting string=w199:string)  [unwired: 2 in, 1 out]
                n108 = Build Array(w202) -> (w201:i32[])
                n109 = Bundle By Name(cluster=w205, "Rt Loop Events"=RT_Loop_Events."Send Reply", "Message Data"=w199, "Data Array"=w201, "error"=errorcluster {"status"=FALSE, "code"=0, "source"=""}) -> (w204:T13)
              }
              frame "xml Get Configuration", "Get Config" {
                n110 = global read "_FW_Sim Global.vi" "Configuration 2"() -> (w206:T4)
                n111 = case shown="\"xml Get Configuration\", Default" w207 {
                  tunnel: w206 -> [w213 w218]
                  tunnel: [w214 w217] -> w209
                  tunnel: [w215 w216] -> w208
                  frame "xml Get Configuration", Default {
                    n112 = call "_Write XML Configuration.vi"("Configuration"=w213) -> ("error out"=w215:errorcluster, "XML String"=w214:string)  [unwired: 1 in, 4 out]
                  }
                  frame "Get Config" {
                    n113 = Flatten To String(anything=w218) -> (data string=w217:string, error out=w216:errorcluster)  [unwired: 1 in, 3 out]
                  }
                }
                n114 = Bundle By Name(cluster=w212, "Rt Loop Events"=RT_Loop_Events."Send Reply", "Message Data"=w209, "error"=w208) -> (w211:T13)
              }
              frame "xml Get Table", "Get Table" {
                # "Get a Calibration/Resolution Table"
                n115 = case shown="\"xml Get Table\", Default" w223 {
                  selector: w223 -> [w231 w236]
                  tunnel: w226 -> [w235 w238]
                  tunnel: [w230 w237] -> w220
                  tunnel: [w231 w236] -> w222
                  frame "xml Get Table", Default {
                    n116 = Unflatten From String(type=0, binary string=w235, data includes array or string size? (T)=FALSE, byte order (0:big-endian, network order)=T16."big-endian, network order") -> (value=w230:i32)  [unwired: 1 in, 2 out]
                  }
                  frame "Get Table" {
                    n117 = Decimal String To Number(string=w238) -> (number=w237:i32)  [unwired: 3 out]
                  }
                }
                n118 = case shown="0, Default" w220 {
                  selector: w220 -> [w245 w247 w249 w251 w253 w255 w257 w259 w261 w263 w265 w267 w269 w271 w273 w275]
                  tunnel: [w244 w246 w248 w250 w252 w254 w256 w258 w260 w262 w264 w266 w268 w270 w272 w274] -> w225
                  tunnel: [w245 w247 w249 w251 w253 w255 w257 w259 w261 w263 w265 w267 w269 w271 w273 w275] -> w221
                  frame 0, Default {
                    n119 = global read "_FW_Sim Global.vi" "Q1 Cal"() -> (w244:dbl[][])
                  }
                  frame 1 {
                    n120 = global read "_FW_Sim Global.vi" "Q2 Cal"() -> (w246:dbl[][])
                  }
                  frame 2 {
                    n121 = global read "_FW_Sim Global.vi" "Q1 -Cal"() -> (w248:dbl[][])
                  }
                  frame 3 {
                    n122 = global read "_FW_Sim Global.vi" "Q2 -Cal"() -> (w250:dbl[][])
                  }
                  frame 4 {
                    n123 = global read "_FW_Sim Global.vi" "Q1 Res Hi"() -> (w252:dbl[][])
                  }
                  frame 5 {
                    n124 = global read "_FW_Sim Global.vi" "Q2 Res Hi"() -> (w254:dbl[][])
                  }
                  frame 6 {
                    n125 = global read "_FW_Sim Global.vi" "Q1 Res Med"() -> (w256:dbl[][])
                  }
                  frame 7 {
                    n126 = global read "_FW_Sim Global.vi" "Q2 Res Med"() -> (w258:dbl[][])
                  }
                  frame 8 {
                    n127 = global read "_FW_Sim Global.vi" "Q1 Res Lo"() -> (w260:dbl[][])
                  }
                  frame 9 {
                    n128 = global read "_FW_Sim Global.vi" "Q2 Res Lo"() -> (w262:dbl[][])
                  }
                  frame 10 {
                    n129 = global read "_FW_Sim Global.vi" "Q1 -Res Lo"() -> (w264:dbl[][])
                  }
                  frame 11 {
                    n130 = global read "_FW_Sim Global.vi" "Q2 -Res Hi"() -> (w266:dbl[][])
                  }
                  frame 12 {
                    n131 = global read "_FW_Sim Global.vi" "Q1 -Res Med"() -> (w268:dbl[][])
                  }
                  frame 13 {
                    n132 = global read "_FW_Sim Global.vi" "Q2 -Res Med"() -> (w270:dbl[][])
                  }
                  frame 14 {
                    n133 = global read "_FW_Sim Global.vi" "Q1 -Res Lo"() -> (w272:dbl[][])
                  }
                  frame 15 {
                    n134 = global read "_FW_Sim Global.vi" "Q2 -Res Lo"() -> (w274:dbl[][])
                  }
                }
                n135 = case shown="\"xml Get Table\", Default" w222 {
                  tunnel: w225 -> [w241 w243]
                  tunnel: [w240 w242] -> w224
                  tunnel: w221 -> [w239 _]
                  frame "xml Get Table", Default {
                    n136 = call "_Write XML Table.vi"("Table Type"=w239, "Table (2D-DBL)"=w241) -> ("XML String"=w240:string)  [unwired: 1 in, 4 out]
                  }
                  frame "Get Table" {
                    n137 = Flatten To String(anything=w243) -> (data string=w242:string)  [unwired: 1 in, 4 out]
                  }
                }
                n138 = Bundle By Name(cluster=w229, "Rt Loop Events"=RT_Loop_Events."Send Reply", "Message Data"=w224, "error"=errorcluster {"status"=FALSE, "code"=0, "source"=""}) -> (w228:T13)
              }
              frame "xml Set Table", "Update Table" {
                # "Update a Calibration/Resolution Table"
                n139 = call "_Read XML Table.vi"("XML String"=w282) -> ("Table Type"=w279:i32, "Table (2D-DBL)"=w278:dbl[][])  [unwired: 1 in, 4 out]
                n140 = case shown="1" w279 {
                  selector: w279 -> [w288 w291 w294 w297 w300 w303 w306 w309 w312 w315 w318 w321 w324 w327 w330 w333]
                  tunnel: ["Cal" ("key") "Cal2" ("key") "Cal3" ("key") "Cal4" ("key") "Res" ("key") "Res2" ("key") "Res3" ("key") "Res4" ("key") "Res5" ("key") "Res6" ("key") "Res7" ("key") "Res8" ("key") "Res9" ("key") "Res10" ("key") "Res11" ("key") "Res12" ("key")] -> w280
                  tunnel: [w288 w291 w294 w297 w300 w303 w306 w309 w312 w315 w318 w321 w324 w327 w330 w333] -> _
                  tunnel: w278 -> [w287 w290 w293 w296 w299 w302 w305 w308 w311 w314 w317 w320 w323 w326 w329 w332]
                  tunnel: [w287 w290 w293 w296 w299 w302 w305 w308 w311 w314 w317 w320 w323 w326 w329 w332] -> w281
                  frame 0, Default {
                    n141 = global write "_FW_Sim Global.vi" "Q1 Cal"(w287) -> ()
                  }
                  frame 1 {
                    n142 = global write "_FW_Sim Global.vi" "Q2 Cal"(w290) -> ()
                  }
                  frame 2 {
                    n143 = global write "_FW_Sim Global.vi" "Q1 -Cal"(w293) -> ()
                  }
                  frame 3 {
                    n144 = global write "_FW_Sim Global.vi" "Q2 -Cal"(w296) -> ()
                  }
                  frame 4 {
                    n145 = global write "_FW_Sim Global.vi" "Q1 Res Hi"(w299) -> ()
                  }
                  frame 5 {
                    n146 = global write "_FW_Sim Global.vi" "Q2 Res Hi"(w302) -> ()
                  }
                  frame 6 {
                    n147 = global write "_FW_Sim Global.vi" "Q1 Res Med"(w305) -> ()
                  }
                  frame 7 {
                    n148 = global write "_FW_Sim Global.vi" "Q2 Res Med"(w308) -> ()
                  }
                  frame 8 {
                    n149 = global write "_FW_Sim Global.vi" "Q1 Res Lo"(w311) -> ()
                  }
                  frame 9 {
                    n150 = global write "_FW_Sim Global.vi" "Q2 Res Lo"(w314) -> ()
                  }
                  frame 10 {
                    n151 = global write "_FW_Sim Global.vi" "Q1 -Res Hi"(w317) -> ()
                  }
                  frame 11 {
                    n152 = global write "_FW_Sim Global.vi" "Q2 -Res Hi"(w320) -> ()
                  }
                  frame 12 {
                    n153 = global write "_FW_Sim Global.vi" "Q1 -Res Med"(w323) -> ()
                  }
                  frame 13 {
                    n154 = global write "_FW_Sim Global.vi" "Q2 -Res Med"(w326) -> ()
                  }
                  frame 14 {
                    n155 = global write "_FW_Sim Global.vi" "Q1 -Res Lo"(w329) -> ()
                  }
                  frame 15 {
                    n156 = global write "_FW_Sim Global.vi" "Q2 -Res Lo"(w332) -> ()
                  }
                }
                n157 = call "_Save RT Table.vi"("Simulation"=TRUE, "Table"=w281, "key"=w280) -> ("error out"=w277:errorcluster)  [unwired: 1 in, 3 out]
                n158 = call <vilib>:"Clear Errors.vi"("error in (no error)"=w277) -> ("error out"=w283:errorcluster)  [unwired: 5 in, 1 out]
                n159 = Bundle By Name(cluster=w286, "Rt Loop Events"=RT_Loop_Events."Send Reply", "error"=w283) -> (w284:T13)
              }
              frame "xml System Status", "Get Detail Status" {
                # "Get Detailed Instrument Status Report"
                n160 = global read "_FW_Sim Global.vi" "Single Source"() -> (w339:bool)
                n161 = Select(t="<Data>\n<SystemStatus>\nInstrument State=Simulation;\nServer State=0;\nLC1 IN=0;\nLC2 IN=0;\nLC1 Out1=1;\nLC1 Out2=0;\nLC2 Out1=1;\nLC2 Out2=0;\nSystem Error=;\nVacuum Gauge=1;\nVacuum Pressure=1164.34;\nVacuum Error=No Error;\nForeline Pressure=-29.22;\nForeline Error=No Error;\nSource 1=ESI;\nNeb Gas1=385.03;\nAux Gas1=313.04;\nCurtain Gas=109.38;\nCC Gas=439.94;\nOut of Gas=0;\nHSID Temp=198.00;\nSource1 Temp=251.00;\nVoltage Output=1;\nExhaust Pressure=3752.31;\nQ2RF HS1 Temp=36.38;\nQ1RF HS1 Temp=40.53;\nM1RF HS1 Temp=37.11;\nQ2RF HS2 Temp=37.35;\nQ1RF HS2 Temp=40.77;\nM1RF HS2 Temp=36.62;\nCorona Current=0.00;\nHTR PS Current=8.23;\nQ1 Tuning DC=-7.15;\nQ2 Tuning DC=-8.26;\nM1RF Tuning DC=-5.58;\nDoor Interlock=1;\n24V=24;\n28V=28;\n-28V=-28;\n60V=59;\n15V=15;\n-15V=-15;\nLens Board 2 +5V=5;\nLens Board 2 -5V=-5;\nLens Board 1 +5V=5;\nLens Board 1 -5V=-5;\nSource Exhaust Valve=1;\n</SystemStatus>\n<Log>\n97:33:2, Starting Up\n97:33:3, Electronics ON\n97:33:11, System Pumping Down\n97:34:28, Roughing Pump Standby\n97:34:28, Turbo Startup\n97:34:31, Turbo Ready\n97:34:34, System Ready\n</Log>\n</Data>", s=w339, f="<Data>\n<SystemStatus>\nInstrument State=Simulation;\nServer State=0;\nLC1 IN=0;\nLC2 IN=0;\nLC1 Out1=1;\nLC1 Out2=0;\nLC2 Out1=1;\nLC2 Out2=0;\nSystem Error=;\nVacuum Gauge=1;\nVacuum Pressure=1164.34;\nVacuum Error=No Error;\nForeline Pressure=-29.22;\nForeline Error=No Error;\nSource 1=ESI;\nSource 2=APCI;\nNeb Gas1=385.03;\nNeb Gas2=0.00;\nAux Gas1=313.04;\nAux Gas2=0.00;\nCurtain Gas=109.38;\nCC Gas=439.94;\nOut of Gas=0;\nHSID Temp=198.00;\nSource1 Temp=251.00;\nSource2 Temp=106.00;\nVoltage Output=1;\nExhaust Pressure=3752.31;\nQ2RF HS1 Temp=36.38;\nQ1RF HS1 Temp=40.53;\nM1RF HS1 Temp=37.11;\nQ2RF HS2 Temp=37.35;\nQ1RF HS2 Temp=40.77;\nM1RF HS2 Temp=36.62;\nCorona Current=0.00;\nHTR PS Current=8.23;\nQ1 Tuning DC=-7.15;\nQ2 Tuning DC=-8.26;\nM1RF Tuning DC=-5.58;\nDoor Interlock=1;\n24V=24;\n28V=28;\n-28V=-28;\n60V=59;\n15V=15;\n-15V=-15;\nLens Board 2 +5V=5;\nLens Board 2 -5V=-5;\nLens Board 1 +5V=5;\nLens Board 1 -5V=-5;\nSource Exhaust Valve=1;\n</SystemStatus>\n<Log>\n97:33:2, Starting Up\n97:33:3, Electronics ON\n97:33:11, System Pumping Down\n97:34:28, Roughing Pump Standby\n97:34:28, Turbo Startup\n97:34:31, Turbo Ready\n97:34:34, System Ready\n</Log>\n</Data>") -> (s? t:f=w336:string)
                n162 = Bundle By Name(cluster=w341, "Rt Loop Events"=RT_Loop_Events."Send Reply", "Message Data"=w336, "error"=errorcluster {"status"=FALSE, "code"=0, "source"=""}) -> (w340:T13)
              }
              frame "xml Set LC Input Logic", "Set CC Input Logics" {
                # "Set contact closure input logics:\nOption    LC1        LC2\n     0        High      High\n     1        Low        High\n     2        High       Low\n     3        Low        Low"
                n163 = Bundle By Name(cluster=w345, "Rt Loop Events"=RT_Loop_Events."Send Reply", "error"=errorcluster {"status"=FALSE, "code"=0, "source"=""}) -> (w344:T13)
              }
              frame Default {
                n164 = Format Into String(format string="Message Type: %s, not recognized by firmware command receiver.", w352) -> (resulting string=w348:string)  [unwired: 2 in, 1 out]
                n165 = call "_Construct Error Cluster.vi"("reason"=w348) -> ()  [unwired: 3 in, 4 out]
                n166 = Bundle By Name(cluster=errorcluster {"status"=FALSE, "code"=0, "source"=""} ("error"), "source"=w348, "status"=TRUE, "code"=7000) -> (w350:errorcluster)
                n167 = Bundle By Name(cluster=w354, "Rt Loop Events"=RT_Loop_Events."Send Reply", "error"=w350) -> (w353:T13)
              }
            }
          }
          frame True {
            # "No command received from the host at this time,\nor the host has been disconnected."
            n168 = case shown="56, 59, 62, 64, 66" w358 {
              tunnel: w361 -> [w365 w373]
              tunnel: [w364 w372] -> w360
              tunnel: w359 -> [_ w369]
              tunnel: w357 -> [w363 _]
              frame 7100.., Default {
                n169 = Bundle By Name(cluster=w365, "error"=w363, "Rt Loop Events"=RT_Loop_Events."Send Reply") -> (w364:T13)
              }
              frame 56, 59, 62, 64, 66 {
                n170 = local read "# Connections"() -> (w370:u8)
                n171 = Greater?(x=w370, y=u8 2) -> (0:w367:bool)
                n172 = case shown="False" w367 {
                  tunnel: w370 -> [w376 _]
                  tunnel: w369 -> [_ w379]
                  tunnel: [RT_Loop_Events."Wait for Command" ("Rt Loop Events") RT_Loop_Events."Wait for Connection" ("Rt Loop Events")] -> w368
                  frame False {
                    n173 = Increment(x=w376) -> (x+1=w374:u8)
                    n174 = local write "# Connections"(w374) -> ()
                  }
                  frame True {
                    n175 = TCP Close Connection(connection ID=w379, abort (F)=TRUE) -> ()  [unwired: 1 in, 2 out]
                    "Connected" <- FALSE ("Connected?")
                  }
                }
                n176 = Wait Until Next ms Multiple(millisecond multiple=u32 380 ("milliseconds to wait")) -> ()  [unwired: 1 out]
                n177 = Bundle By Name(cluster=w373, "Rt Loop Events"=w368) -> (w372:T13)
              }
            }
          }
        }
      }
      frame "Send Reply" {
        w402 = i32[] []  # Data Array
        w401 = errorcluster {"status"=FALSE, "code"=0, "source"=""}  # error
        w403 = ""  # Info
        # "Send a reply back to the host after receiving each command"
        n178 = Unbundle By Name(w390) -> ("Connection ID"=w406:refnum<k5>, "error"=w397:errorcluster, "Sequence Number"=w396:i32, "Command"=w395:T1, "Message Data"=w394:string, "error"=w393:errorcluster, "Data Array"=w391:i32[])
        n179 = case shown="\"xml Start Run\"..\"xml Get Info\"" w395 {
          selector: w395 -> [w422 w429]
          tunnel: w394 -> [w427 w431]
          tunnel: w393 -> [w426 w430]
          tunnel: [w424 w431] -> w386
          tunnel: [w421 w430] -> w392
          tunnel: w391 -> [w425 _]
          tunnel: [w422 w429] -> w387
          frame Default {
            n180 = Bundle By Name(cluster=T18 {"Info"="", "Data Array"=[], "error out"={"status"=FALSE, "code"=0, "source"=""}} ("Data"), "Info"=w427, "error out"=w426, "Data Array"=w425) -> (w423:T18)
            n181 = Flatten To String(anything=w423) -> (data string=w424:string, error out=w421:errorcluster)  [unwired: 3 in, 1 out]
          }
          frame "xml Start Run".."xml Get Info" {
          }
        }
        n182 = Bundle By Name(cluster=T17 {"Packet Signature"="", "Sequence Number"=0, "Command"=enum."Start", "Data Message Size"=0, "Data Message Size"="", "Data Message"="", "Error Message Size"=0, "Error Message Size"="", "Error Message"="", "Checksum"=0, "Error Message"={"status"=FALSE, "code"=0, "source"=""}, "Command ID"=""} ("Packet Info In"), "Sequence Number"=w396, "Command"=w387, "Data Message"=w386, "Error Message"=w392) -> (w398:T17)
        n183 = call "_TCP Msg Write.vi"("RT"=TRUE, "error in"=w397, "Packet Info In"=w398, "connection ID In"=w406) -> ("error out"=w384:errorcluster, "Packet Info In Out"=w385:T17)  [unwired: 1 in, 5 out]
        n184 = Unbundle By Name(w390) -> ("Msgs"=w389:string)
        n185 = case shown="Error" w384 {
          selector: w384 -> [_ w412]
          tunnel: w389 -> [w407 w420]
          tunnel: [w407 w419] -> w388
          tunnel: w385 -> [_ w417]
          frame No Error {
          }
          frame Error {
            w408 = "\r"
            n186 = Unbundle By Name(w417) -> ("Sequence Number"=w415:i32, "Command"=w414:T1, "Data Message Size"=w413:u32)
            n187 = Unbundle By Name(w412) -> ("status"=w411:bool, "code"=w410:i32, "source"=w409:string)
            n188 = Format Into String(format string="Send: #%d\t%s\tMsg \tSize: %d\tError: %s\tError Code: %d\tError Msg: %s", w415, w414, w413, w411, w410, w409) -> (resulting string=w416:string)  [unwired: 2 in, 1 out]
            n189 = Concatenate Strings(w408, w416, w408, w420) -> (w419:string)
          }
        }
        n190 = Bundle By Name(cluster=w390, "Rt Loop Events"=RT_Loop_Events."Wait for Command", "Message Data"=w403, "Data Array"=w402, "error"=w401, "Msgs"=w388) -> (w404:T13)
      }
    }
    n191 = Unbundle By Name(w46) -> ("Msgs"=→"Messages":string)
  }
  n192 = flat-sequence {
    tunnel: w1 -> [_]
    frame #0 {
      n193 = control-ref of="This VI"() -> (w433:refnum<vi>)
      n194 = property class="VI"(reference=w433, "FP.State"=T25."Closed" ("Front Panel Window:State")) -> ()  [unwired: 1 in, 2 out]
    }
  }
